vi "校准UI.vi"() -> ()   [LabVIEW 2016, in "斯坦道多参数.lvlib"]
uses:
  <vilib>/Utility/miscctls.llb/LVPointTypeDef.ctl
  <vilib>/Utility/miscctls.llb/LVPositionTypeDef.ctl
  <vilib>/ptbypt/NI_PtbyPt.lvlib
panel:
  out "溶解氧浓度值":dbl=25.0 caption="检测值：" format="%#.2f mg/L"
  out "电极状态标志":u16
  in  "恢复出厂":bool
  in  "电极系数面板":enum32{"选项卡 1"}(tab)
  out "B":dbl=25.0 caption="电极零点：" format="%#.6f"
  out "K":dbl=25.0 caption="电极系数：" format="%#.6f"
  in  "测试参数面板":enum32{"选项卡 1"}(tab)
  in  "自动盐度补偿":bool caption="自动盐度补偿："
  in  "偏移修正值":dbl=25.0 caption="偏移修正值：" format="%#_6f"
  in  "滤波次数":dbl=25.0 caption="滤波次数：" format="%#_6f"
  in  "测量量程":u16(ring)=1 caption="测量量程："
  in  "盐度":dbl=25.0 caption="盐度：" format="%#_6f"
  in  "大气压力":dbl=25.0 caption="大气压力：" format="%#_6f"
  in  "温度系数":dbl=25.0 caption="温度系数：" format="%#.6f"
  out "信号值":dbl=25.0 caption="信号值：" format="%#.2f mV"
  out "检测值":dbl=25.0 caption="检测值：" format="%#.2f"
  out "序列号":string caption="序列号："
  in  "选项卡控件 3":enum32{"选项卡 1"}(tab)
  in  "清扫间隔":u16=25 caption="清扫间隔："
  in  "清扫次数":u16=25 caption="清扫次数："
  in  "清洗":bool caption="探头清洗："
  in  "清扫模式":u16(ring)=1 caption="清扫模式：" items=["自动", "手动"]
  in  "选项卡控件 2":enum32{"选项卡 1"}(tab)
  in  "温度校准系数写入":bool
  in  "温度校准系数读取":bool
  in  "BT":dbl caption="B：" format="%#.6f"
  in  "KT":dbl=1.0 caption="K：" format="%#.6f"
  in  "实际温度":dbl=25.0 caption="校准温度：" format="%.2f ℃"
  out "当前温度":dbl caption="探头温度：" format="%.2f ℃"
  in  "校准温度":bool
  in  "选项卡控件":enum32{"选项卡 1"}(tab)
  in  "第三点确认校准":bool
  in  "第二点确认校准":bool
  in  "标液一":cluster{"标准值":dbl, "检测值":dbl, "原始值":dbl} caption="标液一：" {"原始值" format="%#_6f"; "检测值" format="%#_6f"; "标准值" format="%#.6f"}
  in  "标液二":cluster{"标准值":dbl, "检测值":dbl, "原始值":dbl} caption="标液二：" {"原始值" format="%#_6f"; "检测值" format="%#_6f"; "标准值" format="%#.6f"}
  in  "标液三":cluster{"标准值":dbl, "检测值":dbl, "原始值":dbl} caption="标液三：" {"原始值" format="%#_6f"; "检测值" format="%#_6f"; "标准值" format="%#.6f"}
  in  "标液一开始校准":bool
  in  "第一点确认校准":bool
  in  "标液二开始校准":bool
  in  "标液三开始校准":bool
  in  "显示曲线":bool
  in  "校准记录":string="校准记录\n---------------------------------------------\n序列号：\n温度值：\n标准值：\n检测值：\n原始值：\n校准时间："
  in  "校准方式":u16(ring)=1 caption="校准方式：" items=["单点校准", "两点校准", "三点校准"]
  in  "校准参数":u16(ring) caption="校准参数：" items=["pH"=0, "DO"=1, "浊度"=2, "电导率"=3, "COD"=7, "氯化物"=9, "氨氮"=10]
  # "检测值"
  # "信号值"
  # "标准值"
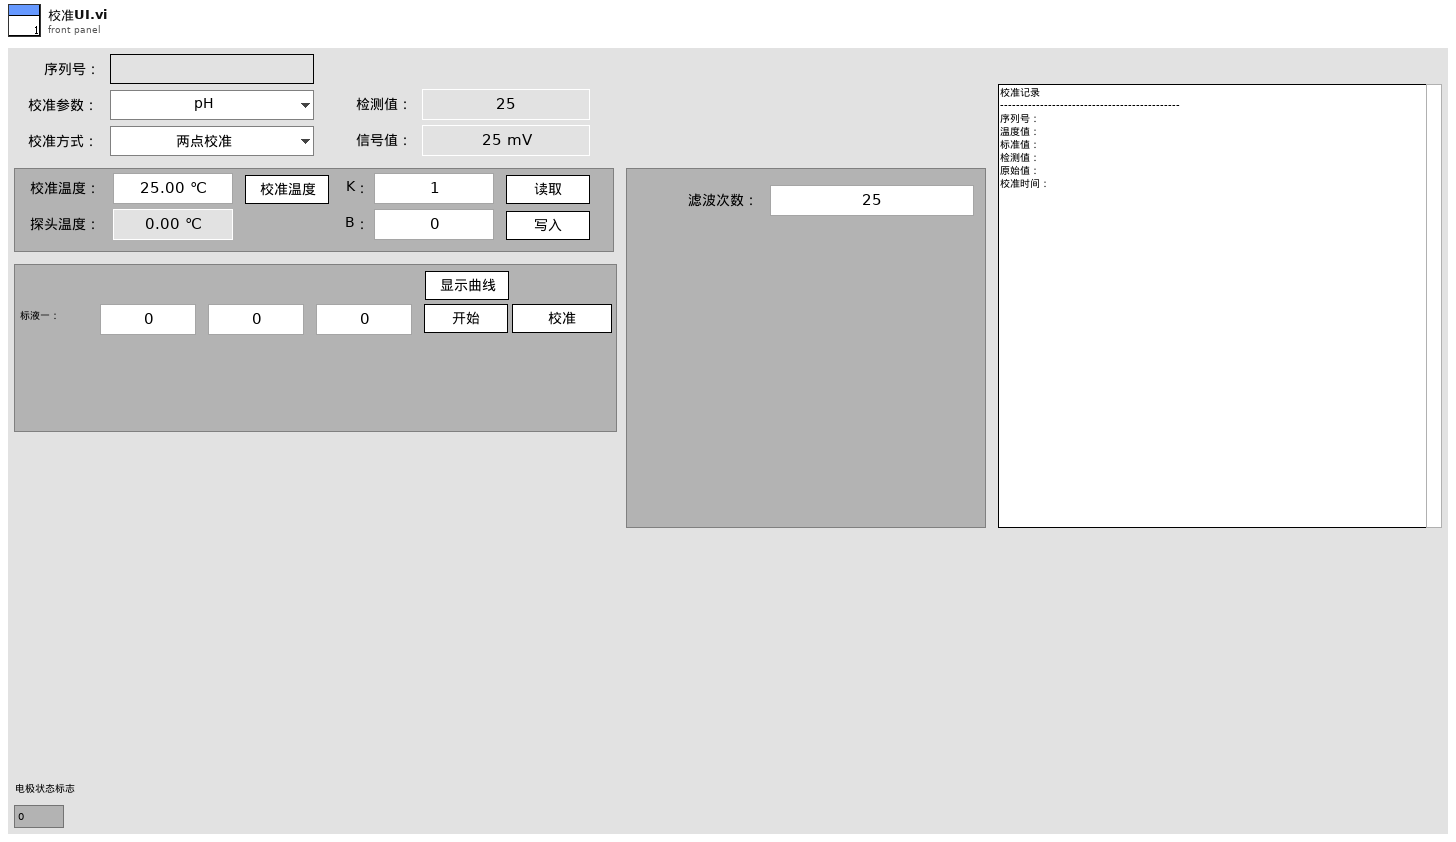
[diagram p1: front panel]
types:
  T1 = typedef "LVPointTypeDef.ctl" = cluster{"Horizontal":i16, "Vertical":i16}
  T2 = cluster{"ph":bool, "DO":bool, "Cond":bool, "Turb":bool, "叶绿素a":bool, "藻密度":bool, "ORP":bool, "COD":bool, "DO2":bool, bool, "氨氮":bool, "水中油":bool}
  T3 = typedef "斯坦道多参数.lvlib/探头类型.ctl" = enum16{"禹山", "国弘", "纳清", "STD"}
  T4 = typedef "LVStringsAndValuesArrayTypeDef_U16.ctl" = cluster{"String":string, "Value":u16}[]
  T5 = enum8{"Enabled", "Disabled", "Disabled and Grayed Out"}
  T6 = typedef "LVPositionTypeDef.ctl" = cluster{"Left":i32, "Top":i32}
  T7 = cluster{"pH":u32, "DO":u32, "Cond":u32, "Turb":u32, "叶绿素a":u32, "藻密度":u32, "ORP":u32, "COD":u32, "氯化物":u32, "氨氮":u32, "水中油":u32}
  T8 = cluster{"电极状态标志":u16, "电极型号标志":u16, "酸碱度测量值":sgl, "温度测量值":sgl, "酸碱度信号值":sgl, "温度信号值":sgl, "酸碱度偏移修正值":sgl, "温度偏移修正值":sgl, "手动温度补偿值":sgl, "酸碱度电极零点":sgl, "酸碱度电极斜率":sgl, "第1点标准值记录":sgl, "第1点信号值记录":sgl, "第1点温度值记录":sgl, "第2点标准值记录":sgl, "第2点信号值记录":sgl, "第2点温度值记录":sgl, "命令滤波设定":u16, "温度模式":enum16{"ATC", "MTC"}, "生产批次":u16, "电极序号":u16, "串口地址":u16, "串口波特率":enum16{"9600", "19200", "115200"}, "串口校验位":enum16{"NONE", "ODD", "EVEN"}, "串口停止位":enum16{"1bit", "2bit"}, "第一点标准值":sgl, "第二点标准值":sgl}
  T9 = cluster{"报警码":u16, "溶解氧数值（mg/L）":sgl, "溶解氧数据（%）":sgl, "温度数据":sgl, "溶解氧原始信号 nA":sgl, "大气压力":sgl, "盐度":sgl, "0X0009_NC":string, "产品名称":string, "序列号":string, "硬件版本":string, "软件版本":string, "通讯地址":u16, "波特率":u16, "设备类型":u16, "0X0026_NC":string, "第一点原始数据":sgl, "第一点校准数据":sgl, "第二点原始数据":sgl, "第二点校准数据":sgl, "探头校准命令":u16, "温度校准参数":sgl, "温度校准命令":u16}
  T10 = cluster{"电极状态标志":u16, "电极型号标志":u16, "溶解氧测量值":sgl, "温度测量值":sgl, "溶解氧饱和度值":sgl, "盐度补偿值":sgl, "大气压补偿值":sgl, "溶解氧偏移修正值":sgl, "温度偏移修正值":sgl, "手动温度补偿值":sgl, "溶解氧电极零点":sgl, "溶解氧电极斜率":sgl, "第1点标准值记录":sgl, "第1点信号值记录":sgl, "第1点温度值记录":sgl, "第2点标准值记录":sgl, "第2点信号值记录":sgl, "第2点温度值记录":sgl, "命令滤波设定":u16, "温度模式":enum16{"ATC", "MTC"}, "生产批次":u16, "电极序号":u16, "串口地址":u16, "串口波特率":enum16{"9600", "19200", "115200"}, "串口校验位":enum16{"NONE", "ODD", "EVEN"}, "串口停止位":enum16{"1bit", "2bit"}, "第一点标准值":sgl, "第二点标准值":sgl}
  T11 = cluster{"电极状态标志":u16, "电极型号标志":u16, "浊度测量值":sgl, "温度测量值":sgl, "浊度信号值":sgl, "浊度偏移修正值":sgl, "温度偏移修正值":sgl, "手动温度补偿值":sgl, "浊度电极零点":sgl, "浊度电极斜率":sgl, "清洁周期":u16, "命令滤波设定":u16, "温度模式":enum16{"ATC", "MTC"}, "生产批次":u16, "电极序号":u16, "串口地址":u16, "串口波特率":enum16{"9600", "19200", "115200"}, "串口校验位":enum16{"NONE", "ODD", "EVEN"}, "串口停止位":enum16{"1bit", "2bit"}, "第一点标准值":sgl, "第二点标准值":sgl, "第三点标准值":sgl}
  T12 = cluster{"报警码":u16, "浊度数值 NTU":sgl, "温度数据":sgl, "原始光强数值":u16, "量程":u16, "平均次数":u16, "清扫模式":u16, "清扫次数":u16, "清扫间隔分钟":u16, "0X000B_NC":string, "产品名称":string, "序列号":string, "硬件版本":string, "软件版本":string, "通讯地址":u16, "波特率":u16, "设备类型":u16, "0X0026_NC":string, "校准量程":u16, "第一点原始光强":u16, "第一点校准数据":sgl, "第二点原始光强":u16, "第二点校准数据":sgl, "第三点原始光强":u16, "第三点校准数据":sgl, "探头校准命令":u16, "温度校准参数":sgl, "温度校准命令":u16}
  T13 = cluster{"电极状态标志":u16, "电极型号标志":u16, "电导率测量值":sgl, "温度测量值":sgl, "电导率信号值":sgl, "温度信号值":sgl, "温度补偿系数":sgl, "电导率偏移修正值":sgl, "温度偏移修正值":sgl, "手动温度补偿值":sgl, "电导率电极零点":sgl, "电导率电极斜率":sgl, "命令滤波设定":u16, "温度模式":enum16{"ATC", "MTC"}, "生产批次":u16, "电极序号":u16, "串口地址":u16, "串口波特率":enum16{"9600", "19200", "115200"}, "串口校验位":enum16{"NONE", "ODD", "EVEN"}, "串口停止位":enum16{"1bit", "2bit"}, "第一点标准值":sgl, "第二点标准值":sgl}
  T14 = cluster{"报警码":u16, "叶绿素a":sgl, "温度数据":sgl, "原始光强数值":u16, "量程":u16, "平均次数":u16, "清扫模式":u16, "清扫次数":u16, "清扫间隔分钟":u16, "0X000B_NC":string, "产品名称":string, "序列号":string, "硬件版本":string, "软件版本":string, "通讯地址":u16, "波特率":u16, "设备类型":u16, "0X0026_NC":string, "校准量程":u16, "第一点原始光强":u16, "第一点校准数据":sgl, "第二点原始光强":u16, "第二点校准数据":sgl, "第三点原始光强":u16, "第三点校准数据":sgl, "探头校准命令":u16, "温度校准参数":sgl, "温度校准命令":u16}
  T15 = cluster{"报警码":u16, "蓝绿藻":sgl, "温度数据":sgl, "原始光强数值":u16, "量程":u16, "平均次数":u16, "清扫模式":u16, "清扫次数":u16, "清扫间隔分钟":u16, "0X000B_NC":string, "产品名称":string, "序列号":string, "硬件版本":string, "软件版本":string, "通讯地址":u16, "波特率":u16, "设备类型":u16, "0X0026_NC":string, "校准量程":u16, "第一点原始光强":u16, "第一点校准数据":sgl, "第二点原始光强":u16, "第二点校准数据":sgl, "第三点原始光强":u16, "第三点校准数据":sgl, "探头校准命令":u16, "温度校准参数":sgl, "温度校准命令":u16}
  T16 = cluster{"电极状态标志":u16, "电极型号标志":u16, "测量值":sgl, "温度测量值":sgl, "信号值":sgl, "温度信号值":sgl, "000AH_NC":sgl, "偏移修正值":sgl, "温度偏移修正值":sgl, "手动温度补偿值":sgl, "命令滤波设定":u16, "温度模式":enum16{"ATC", "MTC"}, "生产批次":u16, "传感器序号":u16, "串口地址":u16, "串口波特率":enum16{"9600", "19200", "115200"}, "串口校验位":enum16{"NONE", "ODD", "EVEN"}, "串口停止位":enum16{"1bit", "2bit"}}
  T17 = cluster{"电极状态标志":u16, "电极型号标志":u16, "COD测量值":sgl, "浊度测量值":sgl, "COD信号值":sgl, "浊度信号值":sgl, "温度测量值":sgl, "COD偏移修正值":sgl, "浊度偏移修正值":sgl, "COD水样校正值":sgl, "温度偏移修正值":sgl, "COD零点系数":sgl, "COD斜率系数":sgl, "浊度零点系数":sgl, "浊度斜率系数":sgl, "COD测值K值":sgl, "浊度测值K值":sgl, "浊度补偿COD系数值":sgl, "COD温度补偿系数值 ":sgl, "测量周期":u16, "清洗周期":u16, "命令寄存器":u16, "数字滤波设定":u16, "温度模式":enum16{"AUTO", "OFF"}, "生产批次":u16, "电极序号":u16, "串口地址":u16, "串口波特率":enum16{"9600", "19200", "115200"}, "串口校验位":enum16{"NONE", "ODD", "EVEN"}, "串口停止位":enum16{"1bit", "2bit"}, "第一点校正指令":u16, "第一点标准值":sgl, "第二点校正指令":u16, "第二点标准值":sgl, "第三点校正指令":u16, "第三点标准值":sgl, "COD吸光度":sgl, "浊度吸光度":sgl, "温度信号值":sgl}
  T18 = cluster{"电极状态标志":u16, "电极型号标志":u16, "测量值":sgl, "温度测量值":sgl, "信号值":sgl, "温度信号值":sgl, "偏移修正值":sgl, "温度偏移修正值":sgl, "手动温度补偿值":sgl, "电极零点":sgl, "电极斜率":sgl, "第1点标准值记录":sgl, "第1点信号值记录":sgl, "第1点温度值记录":sgl, "第2点标准值记录":sgl, "第2点信号值记录":sgl, "第2点温度值记录":sgl, "命令滤波设定":u16, "温度模式":enum16{"ATC", "MTC"}, "生产批次":u16, "电极序号":u16, "串口地址":u16, "串口波特率":enum16{"9600", "19200", "115200"}, "串口校验位":enum16{"NONE", "ODD", "EVEN"}, "串口停止位":enum16{"1bit", "2bit"}, "第一点标准值":sgl, "第二点标准值":sgl}
  T19 = cluster{"电极状态标志":u16, "电极型号标志":u16, "测量值":sgl, "温度测量值":sgl, "信号值":sgl, "水中油B值":sgl, "温度B值":sgl, "水中油零点系数":sgl, "水中油斜率系数":sgl, "水中油K值":sgl, "空白电位值":sgl, "温度信号值":sgl, "温度补偿系数":sgl, "测量档位":u16, "清洁周期":u16, "命令寄存器":u16, "数位滤波设定":u16, "温度模式":enum16{"ATC", "MTC"}, "生产批次":u16, "电极序号":u16, "串口地址":u16, "串口波特率":enum16{"9600", "19200", "115200"}, "串口校验位":enum16{"NONE", "ODD", "EVEN"}, "串口停止位":enum16{"1bit", "2bit"}, "第一点校正指令":u16, "第一点标准值":sgl, "第二点校正指令":u16, "第二点标准值":sgl, "第三点校正指令":u16, "第三点标准值":sgl}
  T20 = enum16{"null", "pH", "DO", "浊度", "电导率", "叶绿素a", "DO2", "藻密度"}
  T21 = enum16{"null", "pH", "DO", "浊度", "电导率", "叶绿素a", "藻密度"}
  T22 = cluster{"禁用":enum8{"Enabled", "Disabled", "Disabled and Grayed Out"}, "禁用 2":enum8{"Enabled", "Disabled", "Disabled and Grayed Out"}, "禁用 3":enum8{"Enabled", "Disabled", "Disabled and Grayed Out"}}
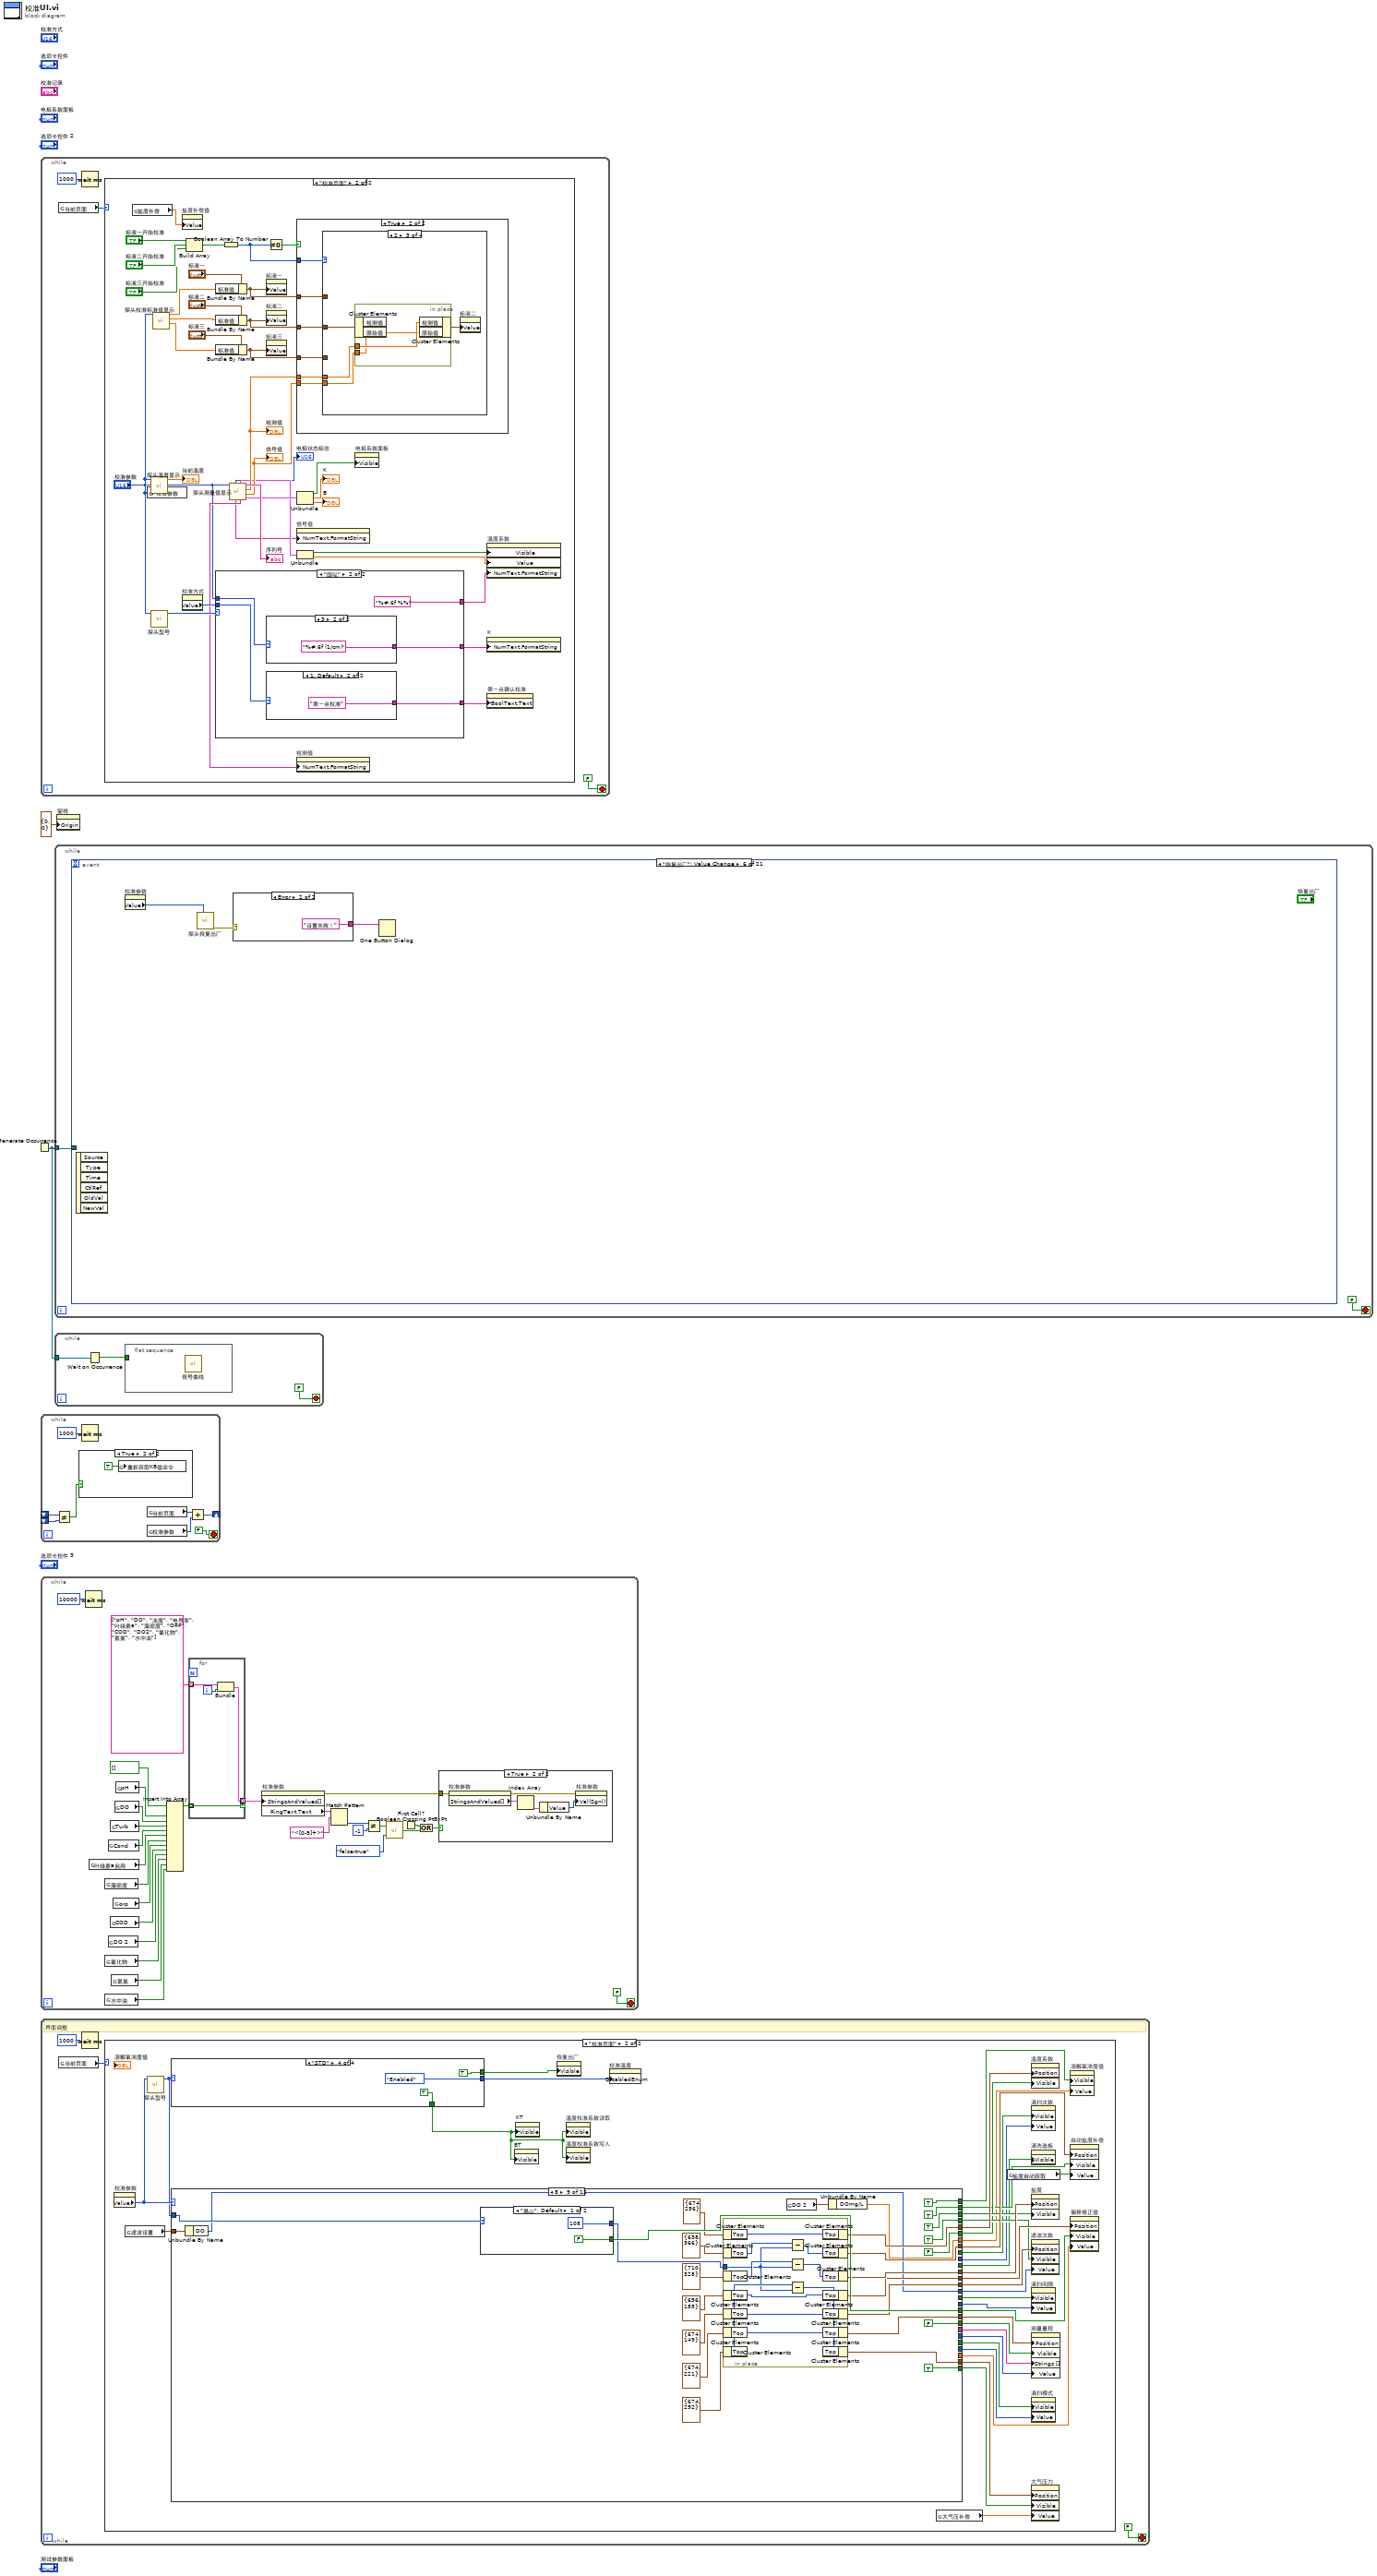
[diagram p0: block diagram]
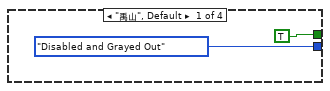
[diagram p4: hidden frame]
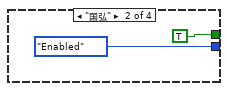
[diagram p5: hidden frame]
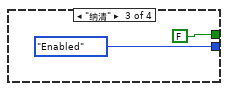
[diagram p6: hidden frame]
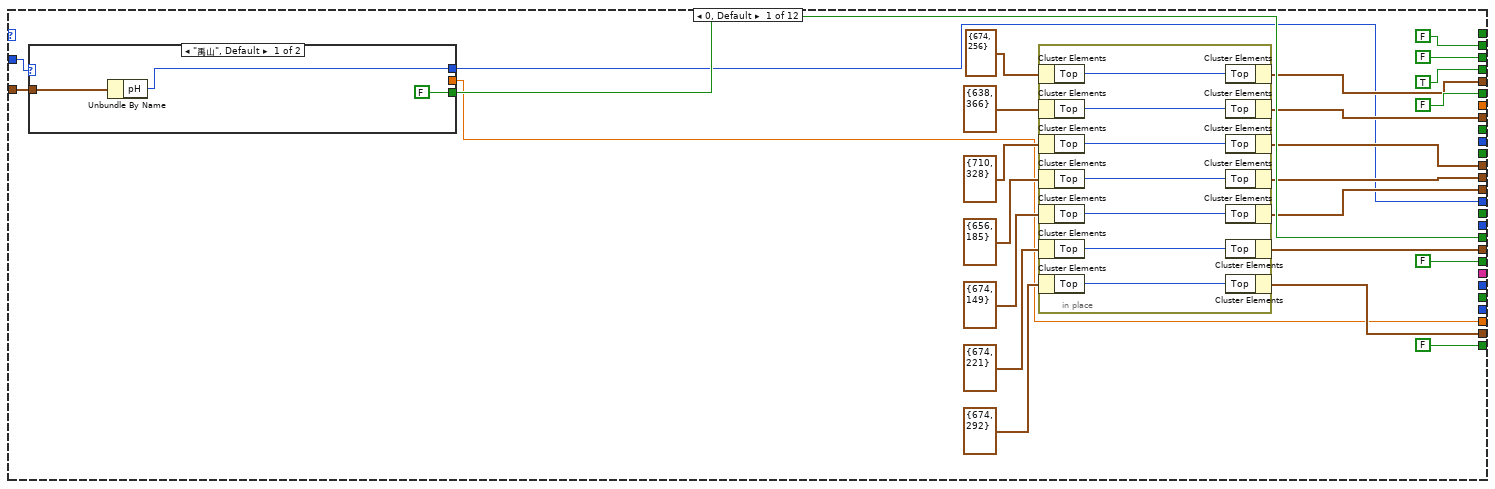
[diagram p7: hidden frame]
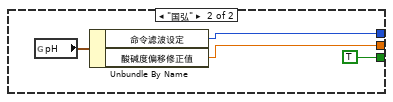
[diagram p8: hidden frame]
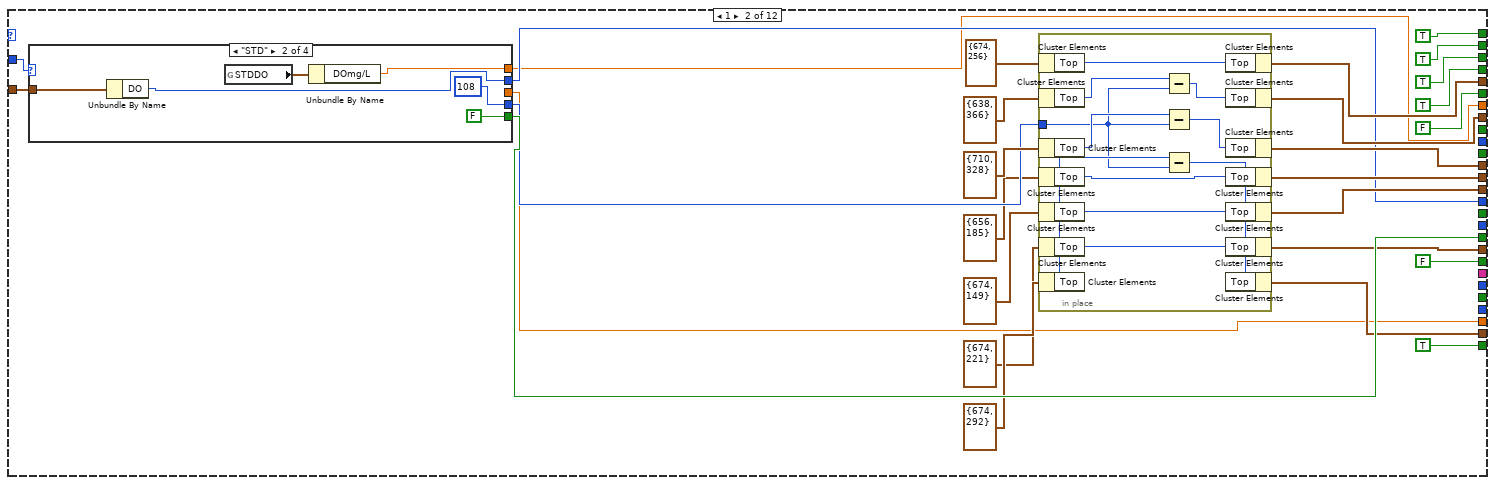
[diagram p9: hidden frame]
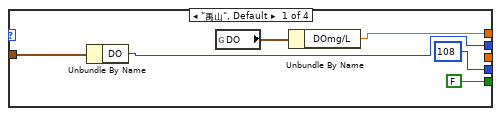
[diagram p10: hidden frame]
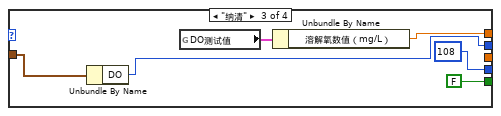
[diagram p11: hidden frame]
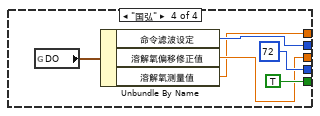
[diagram p12: hidden frame]
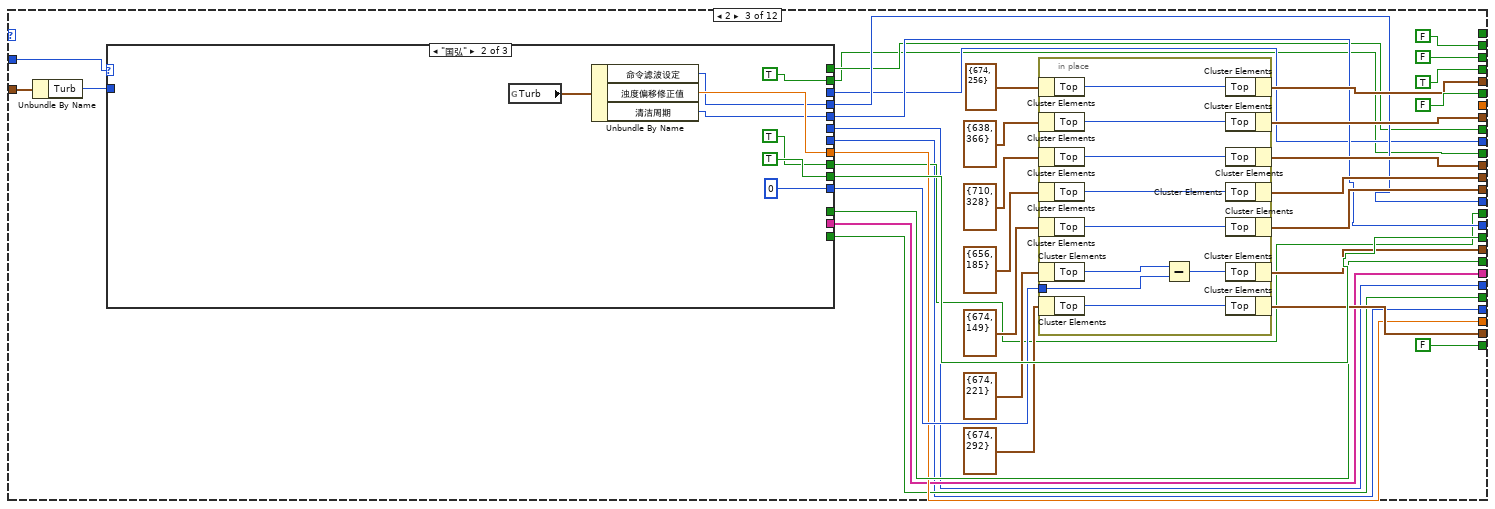
[diagram p13: hidden frame]
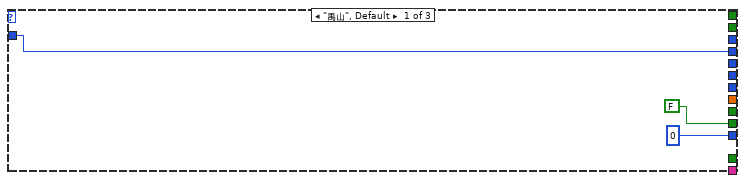
[diagram p14: hidden frame]
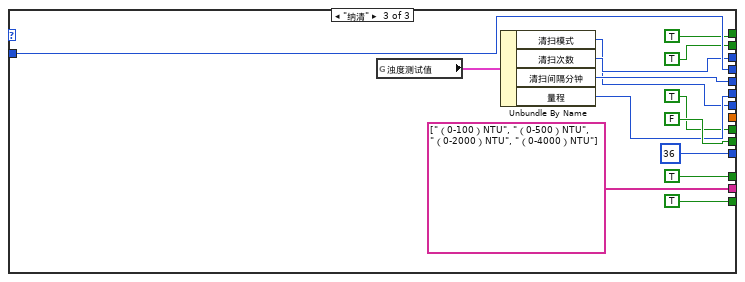
[diagram p15: hidden frame]
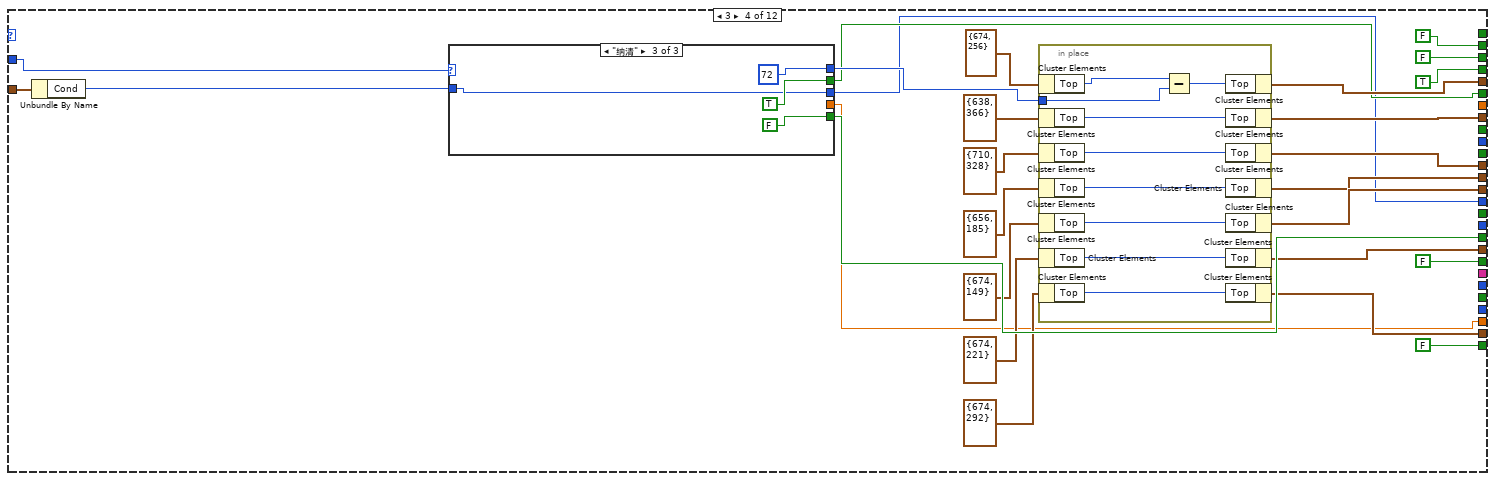
[diagram p16: hidden frame]
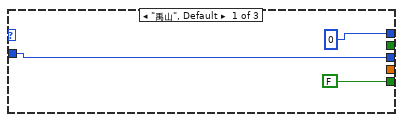
[diagram p17: hidden frame]
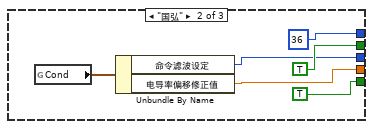
[diagram p18: hidden frame]
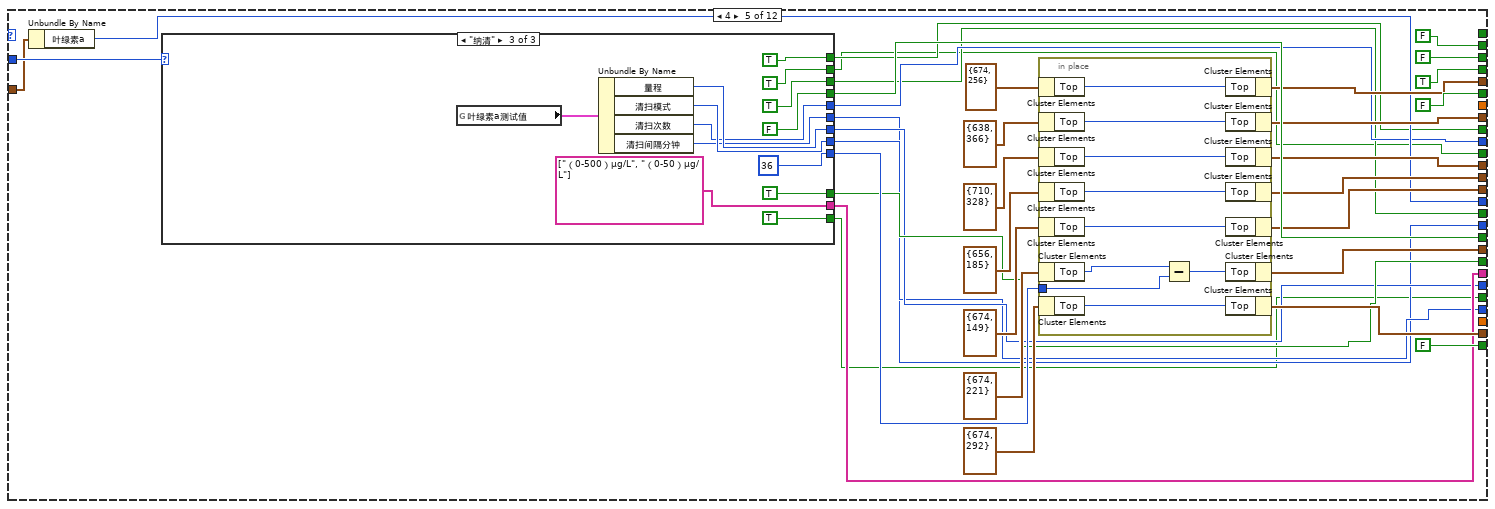
[diagram p19: hidden frame]
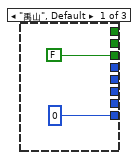
[diagram p20: hidden frame]
diagram:
  n1 = Generate Occurrence() -> (w1:refnum<k4>)
  n2 = while {
    stop <- FALSE stop-if-true
    n3 = global read "多参数全局变量.vi" "当前页面"() -> (w3:enum16{"主页面", "参数页面", "校准页面"})
    n4 = Wait (ms)(milliseconds to wait=u32 1000 ("等待时间（毫秒）")) -> ()  [unwired: 1 out]
    n5 = case shown="\"校准页面\"" w3 {
      frame "主页面", Default {
        n6 = global write "多参数全局变量.vi" "校准运行状态"(T2 {"ph"=FALSE, "DO"=FALSE, "Cond"=FALSE, "Turb"=FALSE, "叶绿素a"=FALSE, "藻密度"=FALSE, "ORP"=FALSE, "COD"=FALSE, "DO2"=FALSE, FALSE, "氨氮"=FALSE, "水中油"=FALSE} ("校准运行状态")) -> ()
      }
      frame "校准页面" {
        n7 = global read "断电保存变量.vi" "盐度补偿"() -> (w29:dbl)
        n8 = global write "多参数全局变量.vi" "校准参数"("校准参数") -> ()
        n9 = call "探头温度显示.vi"("校准参数"="校准参数") -> ("温度数据"=→"当前温度":sgl)  [unwired: 9 in, 1 out]
        n10 = call "探头型号.vi"("校准参数"="校准参数") -> ("探头型号"=w24:T3)  [unwired: 8 in, 2 out]
        n11 = call "探头校准标准值显示.vi"("校准参数"="校准参数") -> ("标液三"=w42:sgl, "标液二"=w41:sgl, "标液一"=w40:sgl)  [unwired: 8 in]
        n12 = property on="盐度补偿值" class="DigNum (strict)"("Value"=w29) -> ()  [unwired: 2 in, 2 out]
        n13 = property on="校准方式" class="Ring (strict)"() -> ("Value"=w22:u16)  [unwired: 2 in, 2 out]
        n14 = Build Array("标液一开始校准", "标液二开始校准", "标液三开始校准") -> (w10:bool[])
        n15 = Bundle By Name(cluster="标液一", "标准值"=w40) -> (w36:cluster{"标准值":dbl, "检测值":dbl, "原始值":dbl})
        n16 = Bundle By Name(cluster="标液二", "标准值"=w41) -> (w35:cluster{"标准值":dbl, "检测值":dbl, "原始值":dbl})
        n17 = Bundle By Name(cluster="标液三", "标准值"=w42) -> (w34:cluster{"标准值":dbl, "检测值":dbl, "原始值":dbl})
        n18 = case shown="\"国弘\"" w24 {
          tunnel: ["校准" w50] -> w23
          tunnel: w22 -> [_ w49]
          tunnel: "校准参数" -> [_ w48]
          tunnel: ["%#.6f" ("数值文本.格式字符串") w47] -> w15
          tunnel: ["%#.6f" ("数值文本.格式字符串") "%#.6f %%" ("数值文本.格式字符串")] -> w14
          frame "禹山", Default {
          }
          frame "国弘" {
            n19 = case shown="3" w48 {
              tunnel: ["%#.6f" ("数值文本.格式字符串") "%#.6f (1/cm)" ("数值文本.格式字符串")] -> w47
              frame 0, Default {
              }
              frame 3 {
              }
            }
            n20 = case shown="1, Default" w49 {
              tunnel: ["校准" "第一点校准"] -> w50
              frame 0 {
              }
              frame 1, Default {
              }
            }
          }
        }
        n21 = Boolean Array To Number(Boolean array=w10) -> (number=w8:u32)
        n22 = call "探头测量值显示.vi"("校准参数"="校准参数") -> ("线性系数"=w28:cluster{bool, "K":sgl, "B":sgl}, "信号值"=w30:sgl, "检测值"=w31:sgl, "序列号"=→"序列号":string, "检测值.格式字符串"=w21:string, "温度补偿系数"=w20:cluster{bool, "温度补偿系数":sgl}, "信号值.格式字符串"=w16:string, "电极状态标志"=→"电极状态标志":u16)  [unwired: 3 in]
        "检测值" <- w31
        "信号值" <- w30
        n23 = property on="标液一" class="Clust (strict)"("Value"=w36) -> ()  [unwired: 2 in, 2 out]
        n24 = property on="标液二" class="Clust (strict)"("Value"=w35) -> ()  [unwired: 2 in, 2 out]
        n25 = property on="标液三" class="Clust (strict)"("Value"=w34) -> ()  [unwired: 2 in, 2 out]
        n26 = Not Equal To 0?(x=w8) -> (x != 0?=w9:bool)
        n27 = case shown="True" w9 {
          tunnel: w36 -> [_ w60]
          tunnel: w35 -> [_ w59]
          tunnel: w34 -> [_ w58]
          tunnel: w30 -> [_ w57]
          tunnel: w31 -> [_ w56]
          tunnel: w8 -> [_ w55]
          frame False {
          }
          frame True {
            n28 = case shown="2" w55 {
              tunnel: w56 -> [_ w63 w70 w76]
              tunnel: w57 -> [_ w62 w69 w75]
              tunnel: w60 -> [_ w64 _ _]
              tunnel: w59 -> [_ _ w67 _]
              tunnel: w58 -> [_ _ _ w73]
              frame Default {
              }
              frame 1 {
                n29 = in-place {
                  in-place-border: w63 -> [w66]
                  in-place-border: w62 -> [w65]
                  n30 = in-place-cluster #1(w64) -> ()  [unwired: 2 out]
                  n31 = in-place-cluster #1("检测值"=w66, "原始值"=w65) -> (w61:cluster{"标准值":dbl, "检测值":dbl, "原始值":dbl})
                }
                n32 = property on="标液一" class="Clust (strict)"("Value"=w61) -> ()  [unwired: 2 in, 2 out]
              }
              frame 2 {
                n33 = in-place {
                  in-place-border: w70 -> [w72]
                  in-place-border: w69 -> [w71]
                  n34 = in-place-cluster #2(w67) -> ()  [unwired: 2 out]
                  n35 = in-place-cluster #2("检测值"=w72, "原始值"=w71) -> (w68:cluster{"标准值":dbl, "检测值":dbl, "原始值":dbl})
                }
                n36 = property on="标液二" class="Clust (strict)"("Value"=w68) -> ()  [unwired: 2 in, 2 out]
              }
              frame 4 {
                n37 = in-place {
                  in-place-border: w76 -> [w78]
                  in-place-border: w75 -> [w77]
                  n38 = in-place-cluster #3(w73) -> ()  [unwired: 2 out]
                  n39 = in-place-cluster #3("检测值"=w78, "原始值"=w77) -> (w74:cluster{"标准值":dbl, "检测值":dbl, "原始值":dbl})
                }
                n40 = property on="标液三" class="Clust (strict)"("Value"=w74) -> ()  [unwired: 2 in, 2 out]
              }
            }
          }
        }
        n41 = Unbundle(w28) -> (w27:bool, "K"=→"K":sgl, "B"=→"B":sgl)
        n42 = property on="信号值" class="DigNum (strict)"("NumText.FormatString"=w16) -> ()  [unwired: 2 in, 2 out]
        n43 = Unbundle(w20) -> (w19:bool, "温度补偿系数"=w18:sgl)
        n44 = property on="检测值" class="DigNum (strict)"("NumText.FormatString"=w21) -> ()  [unwired: 2 in, 2 out]
        n45 = property on="电极系数面板" class="TabCtl (strict)"("Visible"=w27) -> ()  [unwired: 2 in, 2 out]
        n46 = property on="温度系数" class="DigNum (strict)"("Visible"=w19, "Value"=w18, "NumText.FormatString"=w14) -> ()  [unwired: 2 in, 2 out]
        n47 = property on="K" class="DigNum (strict)"("NumText.FormatString"=w15) -> ()  [unwired: 2 in, 2 out]
        n48 = property on="第一点确认校准" class="Bool"("BoolText.Text"=w23) -> ()  [unwired: 2 in, 2 out]
      }
    }
  }
  n49 = while {
    shift-right: [w82] -> _
    shift-left: _ -> [w81]
    shift-left: _ -> [w80]
    stop <- FALSE stop-if-true
    n50 = Not Equal?(x=w81, y=w80) -> (x != y?=w79:bool)
    n51 = case shown="True" w79 {
      frame False {
      }
      frame True {
        n52 = global write "多参数全局变量.vi" "重新获取KB值命令"(TRUE ("重新获取KB值命令")) -> ()
      }
    }
    n53 = Wait (ms)(milliseconds to wait=u32 1000 ("等待时间（毫秒）")) -> ()  [unwired: 1 out]
    n54 = global read "多参数全局变量.vi" "当前页面"() -> (w83:enum16{"主页面", "参数页面", "校准页面"})
    n55 = global read "多参数全局变量.vi" "校准参数"() -> (w84:u16)
    n56 = Add(x=w83, y=w84) -> (x+y=w82:u16)
  }
  n57 = while {
    stop <- FALSE stop-if-true
    n58 = Wait (ms)(milliseconds to wait=u32 10000 ("等待时间（毫秒）")) -> ()  [unwired: 1 out]
    n59 = global read "断电保存变量.vi" "叶绿素a启用"() -> (w110:bool)
    n60 = global read "断电保存变量.vi" "藻密度"() -> (w109:bool)
    n61 = global read "断电保存变量.vi" "氯化物"() -> (w89:bool)
    n62 = global read "断电保存变量.vi" "水中油"() -> (w88:bool)
    n63 = global read "断电保存变量.vi" "Cond"() -> (w111:bool)
    n64 = global read "断电保存变量.vi" "DO 2"() -> (w90:bool)
    n65 = global read "断电保存变量.vi" "Turb"() -> (w112:bool)
    n66 = global read "断电保存变量.vi" "COD"() -> (w91:bool)
    n67 = global read "断电保存变量.vi" "氨氮"() -> (w92:bool)
    n68 = global read "断电保存变量.vi" "orp"() -> (w108:bool)
    n69 = global read "断电保存变量.vi" "DO"() -> (w113:bool)
    n70 = global read "断电保存变量.vi" "pH"() -> (w115:bool)
    n71 = Insert Into Array(array=bool[] [] ("数组"), new element #1=w115, new element #2=w113, new element #3=w112, new element #4=w111, new element #5=w110, new element #6=w109, new element #7=w108, new element #8=w91, new element #9=w90, new element #10=w89, new element #11=w92, new element #12=w88) -> (w105:bool[])  [unwired: 1 in]
    n72 = for {
      tunnel: w105 -> [w121] mode=indexing
      tunnel: string[] ["pH", "DO", "浊度", "电导率", "叶绿素a", "藻密度", "ORP", "COD", "DO2", "氯化物", "氨氮", "水中油"] ("字符串[]") -> [w123] mode=indexing
      tunnel: [w122] -> w102 mode=indexing if=w121
      i -> [w124]
      n73 = Bundle(w123, w124) -> (w122:cluster{string, i32})  [unwired: 1 in]
    }
    n74 = property on="校准参数" class="Ring (strict)"("StringsAndValues[]"=w102) -> (error out=w103:errorcluster, "RingText.Text"=w101:string)  [unwired: 2 in, 1 out]
    n75 = Match Pattern(string=w101, regular expression="<[0-9]+>" ("正则表达式")) -> (offset past match=w99:i32)  [unwired: 1 in, 3 out]
    n76 = Not Equal?(x=w99, y=-1) -> (x != y?=w97:bool)
    n77 = call <vilib>:"Boolean Crossing PtByPt.vi"("direction"=enum16{"either", "false-true", "true-false"}."false-true", "input"=w97) -> ("crossing"=w94:bool)  [unwired: 1 in]
    n78 = First Call?() -> (First Call?: T/F=w95:bool)
    n79 = Or(x=w95, y=w94) -> (x .or. y?=w96:bool)
    n80 = case shown="True" w96 {
      tunnel: w103 -> [_ w120]
      frame False {
      }
      frame True {
        n81 = property on="校准参数" class="Ring (strict)"(error in=w120) -> (error out=w119:errorcluster, "StringsAndValues[]"=w118:T4)  [unwired: 1 in, 1 out]
        n82 = Index Array(array=w118) -> (element=w117:cluster{"String":string, "Value":u16})  [unwired: 1 in]
        n83 = Unbundle By Name(w117) -> ("Value"=w116:u16)
        n84 = property on="校准参数" class="Ring (strict)"(error in=w119, "Val(Sgnl)"=w116) -> ()  [unwired: 1 in, 2 out]
      }
    }
  }
  n85 = while {
    stop <- FALSE stop-if-true
    # "界面调整"
    n86 = global read "多参数全局变量.vi" "当前页面"() -> (w126:enum16{"主页面", "参数页面", "校准页面"})
    n87 = Wait (ms)(milliseconds to wait=u32 1000 ("等待时间（毫秒）")) -> ()  [unwired: 1 out]
    n88 = case shown="\"校准页面\"" w126 {
      frame "主页面", Default {
      }
      frame "校准页面" {
        n89 = property on="校准参数" class="Ring (strict)"() -> ("Value"=w161:u16)  [unwired: 2 in, 2 out]
        n90 = global read "断电保存变量.vi" "滤波设置"() -> (w143:T7)
        n91 = call "探头型号.vi"("校准参数"=w161) -> ("探头型号"=w131:T3)  [unwired: 8 in, 2 out]
        n92 = case shown="\"STD\"" w131 {
          tunnel: [TRUE TRUE FALSE TRUE] -> w130
          tunnel: [T5."Disabled and Grayed Out" ("禁用") T5."Enabled" ("禁用") T5."Enabled" ("禁用") T5."Enabled" ("禁用")] -> w129
          tunnel: [_ _ _ TRUE] -> w128
          frame "禹山", Default {
          }
          frame "国弘" {
          }
          frame "纳清" {
          }
          frame "STD" {
          }
        }
        n93 = case shown="8" w161 {
          tunnel: [w181 w222 w294 w356 w411 w471 w523 w561 w594 w635 w665 w699] -> w162
          tunnel: w131 -> [w189 w231 w303 w365 w420 w480 w531 _ w603 _ _ _]
          tunnel: [w179 w220 w292 w354 w409 w469 w521 w559 w592 w633 w663 w697] -> w160
          tunnel: [w177 w218 w290 w352 w407 w467 w519 w557 w590 w631 w661 w695] -> w159
          tunnel: [w175 w216 w288 w350 w405 w465 w517 w555 w588 w629 w659 w693] -> w158
          tunnel: [w183 w224 w296 w358 w413 w473 w525 w563 w596 w637 w667 w701] -> w157
          tunnel: [w185 w227 w299 w361 w416 w476 w527 w565 w599 w639 w669 w704] -> w156
          tunnel: [w184 w225 w297 w359 w414 w474 w526 w564 w597 w638 w668 w702] -> w155
          tunnel: [TRUE TRUE TRUE TRUE TRUE TRUE TRUE TRUE TRUE TRUE TRUE TRUE] -> w154
          tunnel: [FALSE FALSE w287 FALSE w404 w464 FALSE FALSE FALSE FALSE FALSE _] -> w153
          tunnel: [FALSE TRUE FALSE FALSE FALSE FALSE FALSE FALSE TRUE FALSE FALSE FALSE] -> w152
          tunnel: [FALSE FALSE FALSE w348 FALSE FALSE FALSE FALSE FALSE FALSE FALSE FALSE] -> w151
          tunnel: [w192 w234 w306 w368 w423 w483 w534 TRUE w606 TRUE FALSE TRUE] -> w150
          tunnel: [FALSE TRUE FALSE FALSE FALSE FALSE FALSE FALSE TRUE FALSE FALSE FALSE] -> w149
          tunnel: [FALSE TRUE FALSE FALSE FALSE FALSE FALSE FALSE TRUE FALSE FALSE FALSE] -> w148
          tunnel: [w174 w214 w285 w345 w402 w462 w515 w554 w586 w628 w658 w691] -> w145
          tunnel: [w173 w213 w286 w344 _ _ w516 w553 _ w627 _ w692] -> w144
          tunnel: w143 -> [w172 w215 w284 w347 w403 w463 w514 _ w587 _ w657 _]
          tunnel: [_ _ w282 _ w401 w461 _ _ _ _ _ _] -> w142
          tunnel: [_ _ w281 _ w400 w460 _ _ _ _ _ _] -> w141
          tunnel: [_ _ w280 _ w397 w456 _ _ _ _ _ w690] -> w140
          tunnel: [_ _ w279 _ w394 w454 _ _ _ _ _ TRUE] -> w139
          tunnel: [_ _ w278 _ w395 w453 _ _ _ _ _ _] -> w138
          tunnel: [_ _ w277 _ w396 w455 _ _ _ _ _ _] -> w137
          tunnel: [_ _ w276 _ w398 w457 _ _ _ _ _ _] -> w136
          tunnel: [_ _ w275 _ w399 w458 _ _ _ _ _ _] -> w135
          tunnel: [_ _ w274 _ w393 w459 _ _ _ _ _ TRUE] -> w134
          tunnel: [_ w212 _ _ _ _ _ _ w584 _ _ _] -> w132
          tunnel: [_ TRUE _ _ _ _ _ _ TRUE _ _ _] -> w133
          frame 0, Default {
            n94 = case shown="\"禹山\", Default" w189 {
              tunnel: [FALSE TRUE] -> w192
              tunnel: [w204 w208] -> w174
              tunnel: [_ w207] -> w173
              tunnel: w172 -> [w205 _]
              frame "禹山", Default {
                n95 = Unbundle By Name(w205) -> ("pH"=w204:u32)
              }
              frame "国弘" {
                n96 = global read "国弘过程全局变量.vi" "pH"() -> (w209:T8)
                n97 = Unbundle By Name(w209) -> ("命令滤波设定"=w208:u16, "酸碱度偏移修正值"=w207:sgl)
              }
            }
            n98 = in-place {
              n99 = in-place-cluster #4(T6 {"Left"=674, "Top"=256} ("位置 4")) -> ("Top"=w201:i32)
              n100 = in-place-cluster #5(T6 {"Left"=638, "Top"=366} ("位置 7")) -> ("Top"=w197:i32)
              n101 = in-place-cluster #6(T6 {"Left"=710, "Top"=328} ("位置 6")) -> ("Top"=w198:i32)
              n102 = in-place-cluster #7(T6 {"Left"=656, "Top"=185} ("位置 2")) -> ("Top"=w202:i32)
              n103 = in-place-cluster #8(T6 {"Left"=674, "Top"=149} ("位置")) -> ("Top"=w203:i32)
              n104 = in-place-cluster #9(T6 {"Left"=674, "Top"=221} ("位置 3")) -> ("Top"=w200:i32)
              n105 = in-place-cluster #10(T6 {"Left"=674, "Top"=292} ("位置 5")) -> ("Top"=w199:i32)
              n106 = in-place-cluster #4("Top"=w201) -> (w175:T6)
              n107 = in-place-cluster #5("Top"=w197) -> (w184:T6)
              n108 = in-place-cluster #6("Top"=w198) -> (w185:T6)
              n109 = in-place-cluster #7("Top"=w202) -> (w179:T6)
              n110 = in-place-cluster #8("Top"=w203) -> (w181:T6)
              n111 = in-place-cluster #9("Top"=w200) -> (w177:T6)
              n112 = in-place-cluster #10("Top"=w199) -> (w183:T6)
            }
          }
          frame 1 {
            n113 = case shown="\"STD\"" w231 {
              tunnel: [FALSE FALSE FALSE TRUE] -> w234
              tunnel: [108 ("y") 108 ("y") 108 ("y") 72 ("y")] -> w226
              tunnel: w215 -> [w253 w259 w265 _]
              tunnel: [w252 w258 w264 w269] -> w214
              tunnel: [_ _ _ w270] -> w213
              tunnel: [w250 w256 w262 w268] -> w212
              frame "禹山", Default {
                n114 = Unbundle By Name(w253) -> ("DO"=w252:u32)
                n115 = global read "禹山过程全局变量.vi" "DO"() -> (w251:cluster{"温度测量值":sgl, "DO%":sgl, "DOmg/L":sgl})
                n116 = Unbundle By Name(w251) -> ("DOmg/L"=w250:sgl)
              }
              frame "STD" {
                n117 = Unbundle By Name(w259) -> ("DO"=w258:u32)
                n118 = global read "禹山过程全局变量.vi" "STDDO"() -> (w257:cluster{"温度测量值":sgl, "DO%":sgl, "DOmg/L":sgl})
                n119 = Unbundle By Name(w257) -> ("DOmg/L"=w256:sgl)
              }
              frame "纳清" {
                n120 = Unbundle By Name(w265) -> ("DO"=w264:u32)
                n121 = global read "纳清过程全局变量.vi" "DO测试值"() -> (w263:T9)
                n122 = Unbundle By Name(w263) -> ("溶解氧数值（mg/L）"=w262:sgl)
              }
              frame "国弘" {
                n123 = global read "国弘过程全局变量.vi" "DO"() -> (w271:T10)
                n124 = Unbundle By Name(w271) -> ("命令滤波设定"=w269:u16, "溶解氧偏移修正值"=w270:sgl, "溶解氧测量值"=w268:sgl)
              }
            }
            n125 = in-place {
              in-place-border: w226 -> [w243]
              n126 = in-place-cluster #11(T6 {"Left"=674, "Top"=256} ("位置 4")) -> ("Top"=w240:i32)
              n127 = in-place-cluster #12(T6 {"Left"=638, "Top"=366} ("位置 7")) -> ("Top"=w247:i32)
              n128 = in-place-cluster #13(T6 {"Left"=710, "Top"=328} ("位置 6")) -> ("Top"=w249:i32)
              n129 = in-place-cluster #14(T6 {"Left"=656, "Top"=185} ("位置 2")) -> ("Top"=w241:i32)
              n130 = in-place-cluster #15(T6 {"Left"=674, "Top"=149} ("位置")) -> ("Top"=w242:i32)
              n131 = in-place-cluster #16(T6 {"Left"=674, "Top"=221} ("位置 3")) -> ("Top"=w239:i32)
              n132 = in-place-cluster #17(T6 {"Left"=674, "Top"=292} ("位置 5")) -> ("Top"=w245:i32)
              n133 = Subtract(x=w247, y=w243) -> (x-y=w246:i32)
              n134 = Subtract(x=w249, y=w243) -> (x-y=w248:i32)
              n135 = Subtract(x=w245, y=w243) -> (x-y=w244:i32)
              n136 = in-place-cluster #11("Top"=w240) -> (w216:T6)
              n137 = in-place-cluster #12("Top"=w246) -> (w225:T6)
              n138 = in-place-cluster #13("Top"=w248) -> (w227:T6)
              n139 = in-place-cluster #14("Top"=w241) -> (w220:T6)
              n140 = in-place-cluster #15("Top"=w242) -> (w222:T6)
              n141 = in-place-cluster #16("Top"=w239) -> (w218:T6)
              n142 = in-place-cluster #17("Top"=w244) -> (w224:T6)
            }
          }
          frame 2 {
            n143 = Unbundle By Name(w284) -> ("Turb"=w283:u32)
            n144 = case shown="\"国弘\"" w303 {
              tunnel: [FALSE TRUE FALSE] -> w306
              tunnel: [0 ("y") 0 ("y") 36 ("y")] -> w298
              tunnel: [_ _ TRUE] -> w287
              tunnel: [_ w326 _] -> w286
              tunnel: [w319 w325 w340] -> w285
              tunnel: w283 -> [w319 _ w340]
              tunnel: [_ _ string[] ["（0-100）NTU", "（0-500）NTU", "（0-2000）NTU", "（0-4000）NTU"]] -> w282
              tunnel: [_ _ w337] -> w281
              tunnel: [_ w324 w335] -> w280
              tunnel: [_ TRUE TRUE] -> w279
              tunnel: [_ _ TRUE] -> w278
              tunnel: [_ _ TRUE] -> w277
              tunnel: [_ _ w332] -> w276
              tunnel: [_ _ w331] -> w275
              tunnel: [_ TRUE TRUE] -> w274
              frame "禹山", Default {
              }
              frame "国弘" {
                n145 = global read "国弘过程全局变量.vi" "Turb"() -> (w327:T11)
                n146 = Unbundle By Name(w327) -> ("命令滤波设定"=w325:u16, "浊度偏移修正值"=w326:sgl, "清洁周期"=w324:u16)
              }
              frame "纳清" {
                n147 = global read "纳清过程全局变量.vi" "浊度测试值"() -> (w338:T12)
                n148 = Unbundle By Name(w338) -> ("清扫模式"=w331:u16, "清扫次数"=w332:u16, "清扫间隔分钟"=w335:u16, "量程"=w337:u16)
              }
            }
            n149 = in-place {
              in-place-border: w298 -> [w310]
              n150 = in-place-cluster #18(T6 {"Left"=674, "Top"=256} ("位置 4")) -> ("Top"=w316:i32)
              n151 = in-place-cluster #19(T6 {"Left"=638, "Top"=366} ("位置 7")) -> ("Top"=w313:i32)
              n152 = in-place-cluster #20(T6 {"Left"=710, "Top"=328} ("位置 6")) -> ("Top"=w312:i32)
              n153 = in-place-cluster #21(T6 {"Left"=656, "Top"=185} ("位置 2")) -> ("Top"=w317:i32)
              n154 = in-place-cluster #22(T6 {"Left"=674, "Top"=149} ("位置")) -> ("Top"=w318:i32)
              n155 = in-place-cluster #23(T6 {"Left"=674, "Top"=221} ("位置 3")) -> ("Top"=w315:i32)
              n156 = in-place-cluster #24(T6 {"Left"=674, "Top"=292} ("位置 5")) -> ("Top"=w314:i32)
              n157 = Subtract(x=w315, y=w310) -> (x-y=w311:i32)
              n158 = in-place-cluster #18("Top"=w316) -> (w288:T6)
              n159 = in-place-cluster #19("Top"=w313) -> (w297:T6)
              n160 = in-place-cluster #20("Top"=w312) -> (w299:T6)
              n161 = in-place-cluster #21("Top"=w317) -> (w292:T6)
              n162 = in-place-cluster #22("Top"=w318) -> (w294:T6)
              n163 = in-place-cluster #23("Top"=w311) -> (w290:T6)
              n164 = in-place-cluster #24("Top"=w314) -> (w296:T6)
            }
          }
          frame 3 {
            n165 = Unbundle By Name(w347) -> ("Cond"=w346:u32)
            n166 = case shown="\"纳清\"" w365 {
              tunnel: [FALSE TRUE FALSE] -> w368
              tunnel: [0 ("y") 36 ("y") 72 ("y")] -> w360
              tunnel: [_ TRUE TRUE] -> w348
              tunnel: w346 -> [w380 _ w389]
              tunnel: [w380 w383 w389] -> w345
              tunnel: [_ w384 _] -> w344
              frame "禹山", Default {
              }
              frame "国弘" {
                n167 = global read "国弘过程全局变量.vi" "Cond"() -> (w385:T13)
                n168 = Unbundle By Name(w385) -> ("命令滤波设定"=w383:u16, "电导率偏移修正值"=w384:sgl)
              }
              frame "纳清" {
              }
            }
            n169 = in-place {
              in-place-border: w360 -> [w372]
              n170 = in-place-cluster #25(T6 {"Left"=674, "Top"=256} ("位置 4")) -> ("Top"=w377:i32)
              n171 = in-place-cluster #26(T6 {"Left"=638, "Top"=366} ("位置 7")) -> ("Top"=w375:i32)
              n172 = in-place-cluster #27(T6 {"Left"=710, "Top"=328} ("位置 6")) -> ("Top"=w374:i32)
              n173 = in-place-cluster #28(T6 {"Left"=656, "Top"=185} ("位置 2")) -> ("Top"=w378:i32)
              n174 = in-place-cluster #29(T6 {"Left"=674, "Top"=149} ("位置")) -> ("Top"=w379:i32)
              n175 = in-place-cluster #30(T6 {"Left"=674, "Top"=221} ("位置 3")) -> ("Top"=w371:i32)
              n176 = in-place-cluster #31(T6 {"Left"=674, "Top"=292} ("位置 5")) -> ("Top"=w376:i32)
              n177 = Subtract(x=w377, y=w372) -> (x-y=w373:i32)
              n178 = in-place-cluster #25("Top"=w373) -> (w350:T6)
              n179 = in-place-cluster #26("Top"=w375) -> (w359:T6)
              n180 = in-place-cluster #27("Top"=w374) -> (w361:T6)
              n181 = in-place-cluster #28("Top"=w378) -> (w354:T6)
              n182 = in-place-cluster #29("Top"=w379) -> (w356:T6)
              n183 = in-place-cluster #30("Top"=w371) -> (w352:T6)
              n184 = in-place-cluster #31("Top"=w376) -> (w358:T6)
            }
          }
          frame 4 {
            n185 = Unbundle By Name(w403) -> ("叶绿素a"=w402:u32)
            n186 = case shown="\"纳清\"" w420 {
              tunnel: [FALSE TRUE FALSE] -> w423
              tunnel: [0 ("y") 0 ("y") 36 ("y")] -> w415
              tunnel: [_ _ TRUE] -> w404
              tunnel: [_ _ string[] ["（0-500）μg/L", "（0-50）μg/L"]] -> w401
              tunnel: [_ _ w447] -> w400
              tunnel: [_ _ w446] -> w399
              tunnel: [_ _ w445] -> w398
              tunnel: [_ _ w444] -> w397
              tunnel: [_ _ TRUE] -> w396
              tunnel: [_ _ TRUE] -> w395
              tunnel: [_ _ TRUE] -> w394
              tunnel: [_ _ TRUE] -> w393
              frame "禹山", Default {
              }
              frame "国弘" {
              }
              frame "纳清" {
                n187 = global read "纳清过程全局变量.vi" "叶绿素a测试值"() -> (w448:T14)
                n188 = Unbundle By Name(w448) -> ("量程"=w447:u16, "清扫模式"=w446:u16, "清扫次数"=w445:u16, "清扫间隔分钟"=w444:u16)
              }
            }
            n189 = in-place {
              in-place-border: w415 -> [w427]
              n190 = in-place-cluster #32(T6 {"Left"=674, "Top"=256} ("位置 4")) -> ("Top"=w433:i32)
              n191 = in-place-cluster #33(T6 {"Left"=638, "Top"=366} ("位置 7")) -> ("Top"=w430:i32)
              n192 = in-place-cluster #34(T6 {"Left"=710, "Top"=328} ("位置 6")) -> ("Top"=w429:i32)
              n193 = in-place-cluster #35(T6 {"Left"=656, "Top"=185} ("位置 2")) -> ("Top"=w434:i32)
              n194 = in-place-cluster #36(T6 {"Left"=674, "Top"=149} ("位置")) -> ("Top"=w435:i32)
              n195 = in-place-cluster #37(T6 {"Left"=674, "Top"=221} ("位置 3")) -> ("Top"=w432:i32)
              n196 = in-place-cluster #38(T6 {"Left"=674, "Top"=292} ("位置 5")) -> ("Top"=w431:i32)
              n197 = Subtract(x=w432, y=w427) -> (x-y=w428:i32)
              n198 = in-place-cluster #32("Top"=w433) -> (w405:T6)
              n199 = in-place-cluster #33("Top"=w430) -> (w414:T6)
              n200 = in-place-cluster #34("Top"=w429) -> (w416:T6)
              n201 = in-place-cluster #35("Top"=w434) -> (w409:T6)
              n202 = in-place-cluster #36("Top"=w435) -> (w411:T6)
              n203 = in-place-cluster #37("Top"=w428) -> (w407:T6)
              n204 = in-place-cluster #38("Top"=w431) -> (w413:T6)
            }
          }
          frame 5 {
            n205 = Unbundle By Name(w463) -> ("藻密度"=w462:u32)
            n206 = case shown="\"纳清\"" w480 {
              tunnel: [FALSE TRUE FALSE] -> w483
              tunnel: [0 ("y") 0 ("y") 36 ("y")] -> w475
              tunnel: [_ _ TRUE] -> w464
              tunnel: [_ _ string[] ["（0-2000000）c/mL", "（0-200000）c/mL"]] -> w461
              tunnel: [_ _ w507] -> w460
              tunnel: [_ _ TRUE] -> w459
              tunnel: [_ _ w505] -> w458
              tunnel: [_ _ w504] -> w457
              tunnel: [_ _ w503] -> w456
              tunnel: [_ _ TRUE] -> w455
              tunnel: [_ _ TRUE] -> w454
              tunnel: [_ _ TRUE] -> w453
              frame "禹山", Default {
              }
              frame "国弘" {
              }
              frame "纳清" {
                n207 = global read "纳清过程全局变量.vi" "蓝绿藻测试值"() -> (w508:T15)
                n208 = Unbundle By Name(w508) -> ("量程"=w507:u16, "清扫模式"=w505:u16, "清扫次数"=w504:u16, "清扫间隔分钟"=w503:u16)
              }
            }
            n209 = in-place {
              in-place-border: w475 -> [w487]
              n210 = in-place-cluster #39(T6 {"Left"=674, "Top"=256} ("位置 4")) -> ("Top"=w493:i32)
              n211 = in-place-cluster #40(T6 {"Left"=638, "Top"=366} ("位置 7")) -> ("Top"=w490:i32)
              n212 = in-place-cluster #41(T6 {"Left"=710, "Top"=328} ("位置 6")) -> ("Top"=w489:i32)
              n213 = in-place-cluster #42(T6 {"Left"=656, "Top"=185} ("位置 2")) -> ("Top"=w494:i32)
              n214 = in-place-cluster #43(T6 {"Left"=674, "Top"=149} ("位置")) -> ("Top"=w495:i32)
              n215 = in-place-cluster #44(T6 {"Left"=674, "Top"=221} ("位置 3")) -> ("Top"=w492:i32)
              n216 = in-place-cluster #45(T6 {"Left"=674, "Top"=292} ("位置 5")) -> ("Top"=w491:i32)
              n217 = Subtract(x=w492, y=w487) -> (x-y=w488:i32)
              n218 = in-place-cluster #39("Top"=w493) -> (w465:T6)
              n219 = in-place-cluster #40("Top"=w490) -> (w474:T6)
              n220 = in-place-cluster #41("Top"=w489) -> (w476:T6)
              n221 = in-place-cluster #42("Top"=w494) -> (w469:T6)
              n222 = in-place-cluster #43("Top"=w495) -> (w471:T6)
              n223 = in-place-cluster #44("Top"=w488) -> (w467:T6)
              n224 = in-place-cluster #45("Top"=w491) -> (w473:T6)
            }
          }
          frame 6 {
            n225 = Unbundle By Name(w514) -> ("ORP"=w513:u32)
            n226 = case shown="\"国弘\"" w531 {
              tunnel: [FALSE TRUE] -> w534
              tunnel: [_ w549] -> w516
              tunnel: [w546 w548] -> w515
              tunnel: w513 -> [w546 _]
              frame "禹山", Default {
              }
              frame "国弘" {
                n227 = global read "国弘过程全局变量.vi" "ORP"() -> (w550:T16)
                n228 = Unbundle By Name(w550) -> ("命令滤波设定"=w548:u16, "偏移修正值"=w549:sgl)
              }
            }
            n229 = in-place {
              n230 = in-place-cluster #46(T6 {"Left"=674, "Top"=256} ("位置 4")) -> ("Top"=w543:i32)
              n231 = in-place-cluster #47(T6 {"Left"=638, "Top"=366} ("位置 7")) -> ("Top"=w539:i32)
              n232 = in-place-cluster #48(T6 {"Left"=710, "Top"=328} ("位置 6")) -> ("Top"=w540:i32)
              n233 = in-place-cluster #49(T6 {"Left"=656, "Top"=185} ("位置 2")) -> ("Top"=w544:i32)
              n234 = in-place-cluster #50(T6 {"Left"=674, "Top"=149} ("位置")) -> ("Top"=w545:i32)
              n235 = in-place-cluster #51(T6 {"Left"=674, "Top"=221} ("位置 3")) -> ("Top"=w542:i32)
              n236 = in-place-cluster #52(T6 {"Left"=674, "Top"=292} ("位置 5")) -> ("Top"=w541:i32)
              n237 = in-place-cluster #46("Top"=w543) -> (w517:T6)
              n238 = in-place-cluster #47("Top"=w539) -> (w526:T6)
              n239 = in-place-cluster #48("Top"=w540) -> (w527:T6)
              n240 = in-place-cluster #49("Top"=w544) -> (w521:T6)
              n241 = in-place-cluster #50("Top"=w545) -> (w523:T6)
              n242 = in-place-cluster #51("Top"=w542) -> (w519:T6)
              n243 = in-place-cluster #52("Top"=w541) -> (w525:T6)
            }
          }
          frame 7 {
            n244 = in-place {
              n245 = in-place-cluster #53(T6 {"Left"=674, "Top"=256} ("位置 4")) -> ("Top"=w580:i32)
              n246 = in-place-cluster #54(T6 {"Left"=638, "Top"=366} ("位置 7")) -> ("Top"=w576:i32)
              n247 = in-place-cluster #55(T6 {"Left"=710, "Top"=328} ("位置 6")) -> ("Top"=w577:i32)
              n248 = in-place-cluster #56(T6 {"Left"=656, "Top"=185} ("位置 2")) -> ("Top"=w581:i32)
              n249 = in-place-cluster #57(T6 {"Left"=674, "Top"=149} ("位置")) -> ("Top"=w582:i32)
              n250 = in-place-cluster #58(T6 {"Left"=674, "Top"=221} ("位置 3")) -> ("Top"=w579:i32)
              n251 = in-place-cluster #59(T6 {"Left"=674, "Top"=292} ("位置 5")) -> ("Top"=w578:i32)
              n252 = in-place-cluster #53("Top"=w580) -> (w555:T6)
              n253 = in-place-cluster #54("Top"=w576) -> (w564:T6)
              n254 = in-place-cluster #55("Top"=w577) -> (w565:T6)
              n255 = in-place-cluster #56("Top"=w581) -> (w559:T6)
              n256 = in-place-cluster #57("Top"=w582) -> (w561:T6)
              n257 = in-place-cluster #58("Top"=w579) -> (w557:T6)
              n258 = in-place-cluster #59("Top"=w578) -> (w563:T6)
            }
            n259 = global read "国弘过程全局变量.vi" "COD"() -> (w552:T17)
            n260 = Unbundle By Name(w552) -> ("数字滤波设定"=w554:u16, "COD偏移修正值"=w553:sgl)
          }
          frame 8 {
            n261 = Unbundle By Name(w587) -> ("DO"=w586:u32)
            n262 = case shown="\"禹山\", Default" w603 {
              tunnel: [FALSE TRUE] -> w606
              tunnel: [108 ("y") 72 ("y")] -> w598
              frame "禹山", Default {
              }
              frame "国弘" {
              }
            }
            n263 = in-place {
              in-place-border: w598 -> [w615]
              n264 = in-place-cluster #60(T6 {"Left"=674, "Top"=256} ("位置 4")) -> ("Top"=w612:i32)
              n265 = in-place-cluster #61(T6 {"Left"=638, "Top"=366} ("位置 7")) -> ("Top"=w619:i32)
              n266 = in-place-cluster #62(T6 {"Left"=710, "Top"=328} ("位置 6")) -> ("Top"=w621:i32)
              n267 = in-place-cluster #63(T6 {"Left"=656, "Top"=185} ("位置 2")) -> ("Top"=w613:i32)
              n268 = in-place-cluster #64(T6 {"Left"=674, "Top"=149} ("位置")) -> ("Top"=w614:i32)
              n269 = in-place-cluster #65(T6 {"Left"=674, "Top"=221} ("位置 3")) -> ("Top"=w611:i32)
              n270 = in-place-cluster #66(T6 {"Left"=674, "Top"=292} ("位置 5")) -> ("Top"=w617:i32)
              n271 = Subtract(x=w619, y=w615) -> (x-y=w618:i32)
              n272 = Subtract(x=w621, y=w615) -> (x-y=w620:i32)
              n273 = Subtract(x=w617, y=w615) -> (x-y=w616:i32)
              n274 = in-place-cluster #60("Top"=w612) -> (w588:T6)
              n275 = in-place-cluster #61("Top"=w618) -> (w597:T6)
              n276 = in-place-cluster #62("Top"=w620) -> (w599:T6)
              n277 = in-place-cluster #63("Top"=w613) -> (w592:T6)
              n278 = in-place-cluster #64("Top"=w614) -> (w594:T6)
              n279 = in-place-cluster #65("Top"=w611) -> (w590:T6)
              n280 = in-place-cluster #66("Top"=w616) -> (w596:T6)
            }
            n281 = global read "禹山过程全局变量.vi" "DO 2"() -> (w585:cluster{"温度测量值":sgl, "DO%":sgl, "DOmg/L":sgl})
            n282 = Unbundle By Name(w585) -> ("DOmg/L"=w584:sgl)
          }
          frame 9 {
            n283 = in-place {
              n284 = in-place-cluster #67(T6 {"Left"=674, "Top"=256} ("位置 4")) -> ("Top"=w654:i32)
              n285 = in-place-cluster #68(T6 {"Left"=638, "Top"=366} ("位置 7")) -> ("Top"=w650:i32)
              n286 = in-place-cluster #69(T6 {"Left"=710, "Top"=328} ("位置 6")) -> ("Top"=w651:i32)
              n287 = in-place-cluster #70(T6 {"Left"=656, "Top"=185} ("位置 2")) -> ("Top"=w655:i32)
              n288 = in-place-cluster #71(T6 {"Left"=674, "Top"=149} ("位置")) -> ("Top"=w656:i32)
              n289 = in-place-cluster #72(T6 {"Left"=674, "Top"=221} ("位置 3")) -> ("Top"=w653:i32)
              n290 = in-place-cluster #73(T6 {"Left"=674, "Top"=292} ("位置 5")) -> ("Top"=w652:i32)
              n291 = in-place-cluster #67("Top"=w654) -> (w629:T6)
              n292 = in-place-cluster #68("Top"=w650) -> (w638:T6)
              n293 = in-place-cluster #69("Top"=w651) -> (w639:T6)
              n294 = in-place-cluster #70("Top"=w655) -> (w633:T6)
              n295 = in-place-cluster #71("Top"=w656) -> (w635:T6)
              n296 = in-place-cluster #72("Top"=w653) -> (w631:T6)
              n297 = in-place-cluster #73("Top"=w652) -> (w637:T6)
            }
            n298 = global read "国弘过程全局变量.vi" "氯化物"() -> (w626:T18)
            n299 = Unbundle By Name(w626) -> ("命令滤波设定"=w628:u16, "偏移修正值"=w627:sgl)
          }
          frame 10 {
            n300 = Unbundle By Name(w657) -> ("氨氮"=w658:u32)
            n301 = in-place {
              n302 = in-place-cluster #74(T6 {"Left"=674, "Top"=256} ("位置 4")) -> ("Top"=w684:i32)
              n303 = in-place-cluster #75(T6 {"Left"=638, "Top"=366} ("位置 7")) -> ("Top"=w680:i32)
              n304 = in-place-cluster #76(T6 {"Left"=710, "Top"=328} ("位置 6")) -> ("Top"=w681:i32)
              n305 = in-place-cluster #77(T6 {"Left"=656, "Top"=185} ("位置 2")) -> ("Top"=w685:i32)
              n306 = in-place-cluster #78(T6 {"Left"=674, "Top"=149} ("位置")) -> ("Top"=w686:i32)
              n307 = in-place-cluster #79(T6 {"Left"=674, "Top"=221} ("位置 3")) -> ("Top"=w683:i32)
              n308 = in-place-cluster #80(T6 {"Left"=674, "Top"=292} ("位置 5")) -> ("Top"=w682:i32)
              n309 = in-place-cluster #74("Top"=w684) -> (w659:T6)
              n310 = in-place-cluster #75("Top"=w680) -> (w668:T6)
              n311 = in-place-cluster #76("Top"=w681) -> (w669:T6)
              n312 = in-place-cluster #77("Top"=w685) -> (w663:T6)
              n313 = in-place-cluster #78("Top"=w686) -> (w665:T6)
              n314 = in-place-cluster #79("Top"=w683) -> (w661:T6)
              n315 = in-place-cluster #80("Top"=w682) -> (w667:T6)
            }
          }
          frame 11 {
            n316 = global read "国弘过程全局变量.vi" "水中油"() -> (w687:T19)
            n317 = Unbundle By Name(w687) -> ("数位滤波设定"=w691:u16, "水中油B值"=w692:sgl, "清洁周期"=w690:u16)
            n318 = in-place {
              in-place-border: 0 ("y") -> [w714]
              n319 = in-place-cluster #81(T6 {"Left"=674, "Top"=256} ("位置 4")) -> ("Top"=w720:i32)
              n320 = in-place-cluster #82(T6 {"Left"=638, "Top"=366} ("位置 7")) -> ("Top"=w717:i32)
              n321 = in-place-cluster #83(T6 {"Left"=710, "Top"=328} ("位置 6")) -> ("Top"=w716:i32)
              n322 = in-place-cluster #84(T6 {"Left"=656, "Top"=185} ("位置 2")) -> ("Top"=w721:i32)
              n323 = in-place-cluster #85(T6 {"Left"=674, "Top"=149} ("位置")) -> ("Top"=w722:i32)
              n324 = in-place-cluster #86(T6 {"Left"=674, "Top"=221} ("位置 3")) -> ("Top"=w719:i32)
              n325 = in-place-cluster #87(T6 {"Left"=674, "Top"=292} ("位置 5")) -> ("Top"=w718:i32)
              n326 = Subtract(x=w719, y=w714) -> (x-y=w715:i32)
              n327 = in-place-cluster #81("Top"=w720) -> (w693:T6)
              n328 = in-place-cluster #82("Top"=w717) -> (w702:T6)
              n329 = in-place-cluster #83("Top"=w716) -> (w704:T6)
              n330 = in-place-cluster #84("Top"=w721) -> (w697:T6)
              n331 = in-place-cluster #85("Top"=w722) -> (w699:T6)
              n332 = in-place-cluster #86("Top"=w715) -> (w695:T6)
              n333 = in-place-cluster #87("Top"=w718) -> (w701:T6)
            }
          }
        }
        n334 = property on="BT" class="DigNum (strict)"("Visible"=w128) -> ()  [unwired: 2 in, 2 out]
        n335 = property on="KT" class="DigNum (strict)"("Visible"=w128) -> ()  [unwired: 2 in, 2 out]
        n336 = property on="恢复出厂" class="Bool"("Visible"=w130) -> ()  [unwired: 2 in, 2 out]
        n337 = property on="温度校准系数读取" class="Bool"("Visible"=w128) -> ()  [unwired: 2 in, 2 out]
        n338 = property on="温度校准系数写入" class="Bool"("Visible"=w128) -> ()  [unwired: 2 in, 2 out]
        n339 = property on="校准温度" class="Bool"("DisabledEnum"=w129) -> ()  [unwired: 2 in, 2 out]
        n340 = global read "断电保存变量.vi" "大气压补偿"() -> (w147:dbl)
        n341 = global read "断电保存变量.vi" "盐度自动获取"() -> (w146:bool)
        n342 = property on="温度系数" class="DigNum (strict)"("Position"=w158, "Visible"=w151) -> ()  [unwired: 2 in, 2 out]
        n343 = property on="清扫次数" class="DigNum (strict)"("Visible"=w138, "Value"=w136) -> ()  [unwired: 2 in, 2 out]
        n344 = property on="清洗选板" class="TabCtl (strict)"("Visible"=w134) -> ()  [unwired: 2 in, 2 out]
        n345 = property on="盐度" class="DigNum (strict)"("Position"=w156, "Visible"=w152) -> ()  [unwired: 2 in, 2 out]
        n346 = property on="滤波次数" class="DigNum (strict)"("Position"=w162, "Visible"=w154, "Value"=w145) -> ()  [unwired: 2 in, 2 out]
        n347 = property on="清扫间隔" class="DigNum (strict)"("Visible"=w139, "Value"=w140) -> ()  [unwired: 2 in, 2 out]
        n348 = property on="测量量程" class="Ring (strict)"("Position"=w159, "Visible"=w153, "Strings []"=w142, "Value"=w141) -> ()  [unwired: 2 in, 2 out]
        n349 = property on="清扫模式" class="Ring (strict)"("Visible"=w137, "Value"=w135) -> ()  [unwired: 2 in, 2 out]
        n350 = property on="大气压力" class="DigNum (strict)"("Position"=w157, "Visible"=w148, "Value"=w147) -> ()  [unwired: 2 in, 2 out]
        n351 = property on="溶解氧浓度值" class="DigNum (strict)"("Visible"=w133, "Value"=w132) -> ()  [unwired: 2 in, 2 out]
        n352 = property on="自动盐度补偿" class="Bool (strict)"("Position"=w155, "Visible"=w149, "Value"=w146) -> ()  [unwired: 2 in, 2 out]
        n353 = property on="偏移修正值" class="DigNum (strict)"("Position"=w160, "Visible"=w150, "Value"=w144) -> ()  [unwired: 2 in, 2 out]
      }
    }
  }
  n354 = while {
    tunnel: w1 -> [w723]
    stop <- FALSE stop-if-true
    n355 = event shown="[5] \"恢复出厂\": Value Change" {
      selector: _ -> [_ _ _ _ _ _ _ _ _ _ _ _ _ _ _ _ _ _ _ _ _]
      dyn-events: _ -> [_ _ _ _ _ _ _ _ _ _ _ _ _ _ _ _ _ _ _ _ _]
      timeout: _ -> [_ _ _ _ _ _ _ _ _ _ _ _ _ _ _ _ _ _ _ _ _]
      tunnel: w723 -> [_ _ _ w761 _ _ _ _ _ _ _ _ _ _ _ _ _ _ _ _ _]
      event Timeout {
        n356 = event-data() -> ()  [unwired: 1 in, 3 out]
      }
      event "温度校准系数读取": Value Change {
        n357 = event-data() -> ()  [unwired: 1 in, 6 out]
        n358 = local read "校准参数"() -> (w725:u16)
        n359 = case shown="6" w725 {
          tunnel: [T20."null" ("探头") T20."pH" ("探头") T20."DO" ("探头") T20."浊度" ("探头") T20."电导率" ("探头") T20."叶绿素a" ("探头") T20."DO2" ("探头") T20."藻密度" ("探头")] -> w726
          frame Default {
          }
          frame 0 {
          }
          frame 1 {
          }
          frame 2 {
          }
          frame 3 {
          }
          frame 4 {
          }
          frame 5 {
          }
          frame 6 {
          }
        }
        n360 = global read "多参数全局变量.vi" "MB session in"() -> (w727:refnum<class "MB_Master.lvclass">)
        n361 = call "STD获取温度校准参数.vi"("探头"=w726, "MB session in"=w727) -> ("error out"=w728:errorcluster, "输出值"=w732:cluster{"K":sgl, "B":sgl})  [unwired: 7 in, 1 out]
        n362 = case shown="No Error" w728 {
          tunnel: ["读取成功！" "读取失败！"] -> w729
          frame No Error {
          }
          frame Error {
          }
        }
        n363 = Unbundle By Name(w732) -> ("K"=w731:sgl, "B"=w730:sgl)
        n364 = local write "KT"(w731) -> ()
        n365 = local write "BT"(w730) -> ()
        n366 = One Button Dialog(message=w729) -> ()  [unwired: 1 in, 1 out]
      }
      event "温度校准系数写入": Value Change {
        n367 = event-data() -> ()  [unwired: 1 in, 6 out]
        n368 = local read "校准参数"() -> (w745:u16)
        n369 = case shown="6" w745 {
          tunnel: [T20."null" ("探头") T20."pH" ("探头") T20."DO" ("探头") T20."浊度" ("探头") T20."电导率" ("探头") T20."叶绿素a" ("探头") T20."DO2" ("探头") T20."藻密度" ("探头")] -> w746
          frame Default {
          }
          frame 0 {
          }
          frame 1 {
          }
          frame 2 {
          }
          frame 3 {
          }
          frame 4 {
          }
          frame 5 {
          }
          frame 6 {
          }
        }
        n370 = global read "多参数全局变量.vi" "MB session in"() -> (w747:refnum<class "MB_Master.lvclass">)
        n371 = Bundle("KT"="KT", "BT"="BT") -> (w748:cluster{"KT":dbl, "BT":dbl})  [unwired: 1 in]
        n372 = call "STD设置温度校准参数.vi"("探头"=w746, "用户校准参数"=w748, "MB session in"=w747) -> ("error out"=w744:errorcluster)  [unwired: 7 in, 1 out]
        n373 = case shown="Error" w744 {
          tunnel: ["写入成功！" "写入失败！"] -> w743
          frame No Error {
          }
          frame Error {
          }
        }
        n374 = One Button Dialog(message=w743) -> ()  [unwired: 1 in, 1 out]
      }
      event "显示曲线": Value Change {
        n375 = event-data() -> ()  [unwired: 1 in, 6 out]
        n376 = Set Occurrence(w761) -> ()
      }
      event "温度系数": Value Change {
        n377 = event-data() -> ()  [unwired: 1 in, 6 out]
        n378 = property on="校准参数" class="Ring (strict)"() -> ("Value"=w765:u16)  [unwired: 2 in, 2 out]
        n379 = call "探头温度系数.vi"("校准参数"=w765, "温度系数"="温度系数") -> ("error out"=w762:errorcluster)  [unwired: 9 in]
        n380 = case shown="Error" w762 {
          tunnel: ["设置成功！" "设置失败！"] -> w763
          frame No Error {
          }
          frame Error {
          }
        }
        n381 = One Button Dialog(message=w763) -> ()  [unwired: 1 in, 1 out]
      }
      event "恢复出厂": Value Change {
        n382 = event-data() -> ()  [unwired: 1 in, 6 out]
        n383 = property on="校准参数" class="Ring (strict)"() -> ("Value"=w770:u16)  [unwired: 2 in, 2 out]
        n384 = call "探头恢复出厂.vi"("校准参数"=w770) -> ("error out"=w768:errorcluster)  [unwired: 10 in]
        n385 = case shown="Error" w768 {
          tunnel: ["设置成功！" "设置失败！"] -> w769
          frame No Error {
          }
          frame Error {
          }
        }
        n386 = One Button Dialog(message=w769) -> ()  [unwired: 1 in, 1 out]
      }
      event "测量量程": Value Change {
        n387 = event-data() -> ()  [unwired: 1 in, 6 out]
        n388 = property on="校准参数" class="Ring (strict)"() -> ("Value"=w775:u16)  [unwired: 2 in, 2 out]
        n389 = call "探头校准量程设置.vi"("校准参数"=w775, "校准量程"="测量量程") -> ("error out"=w774:errorcluster)  [unwired: 9 in]
        n390 = call "探头测量量程设置.vi"("校准参数"=w775, "error in (no error)"=w774, "测量量程设置"="测量量程") -> ("error out"=w776:errorcluster)  [unwired: 8 in]
        n391 = case shown="Error" w776 {
          tunnel: ["设置成功！" "设置失败！"] -> w777
          frame No Error {
          }
          frame Error {
          }
        }
        n392 = One Button Dialog(message=w777) -> ()  [unwired: 1 in, 1 out]
      }
      event "自动盐度补偿", "大气压力", "盐度", "滤波次数": Value Change {
        n393 = event-data() -> ()  [unwired: 1 in, 6 out]
        n394 = flat-sequence {
          tunnel: [w781] -> w780
          tunnel: w780 -> [_]
          frame #0 {
            n395 = property on="校准参数" class="Ring (strict)"() -> ("Value"=w783:u16)  [unwired: 2 in, 2 out]
            n396 = global write "断电保存变量.vi" "盐度补偿"("盐度") -> ()
            n397 = global write "断电保存变量.vi" "大气压补偿"("大气压力") -> ()
            n398 = call "探头滤波次数.vi"("校准参数"=w783, "滤波次数"="滤波次数") -> ("error out"=w781:errorcluster)  [unwired: 9 in]
            n399 = global write "断电保存变量.vi" "盐度自动获取"("自动盐度补偿") -> ()
          }
          frame #1 {
            n400 = call "配置文件保存.vi"() -> ()  [unwired: 12 in]
          }
        }
      }
      event "清洗": Value Change {
        n401 = event-data() -> ()  [unwired: 1 in, 6 out]
        n402 = property on="校准参数" class="Ring (strict)"() -> ("Value"=w787:u16)  [unwired: 2 in, 2 out]
        n403 = call "探头手动清洗.vi"("校准参数"=w787) -> ("error out"=w788:errorcluster)  [unwired: 10 in]
        n404 = case shown="No Error" w788 {
          tunnel: ["启动成功！" "启动失败！"] -> w789
          frame No Error {
          }
          frame Error {
          }
        }
        n405 = One Button Dialog(message=w789) -> ()  [unwired: 1 in, 1 out]
      }
      event "清扫模式": Value Change {
        n406 = event-data() -> ()  [unwired: 1 in, 6 out]
        n407 = property on="校准参数" class="Ring (strict)"() -> ("Value"=w793:u16)  [unwired: 2 in, 2 out]
        n408 = case shown="5" w793 {
          tunnel: [T21."null" ("探头") T21."pH" ("探头") T21."DO" ("探头") T21."浊度" ("探头") T21."电导率" ("探头") T21."叶绿素a" ("探头") T21."藻密度" ("探头") 17] -> w792
          frame Default {
          }
          frame 0 {
          }
          frame 1 {
          }
          frame 2 {
          }
          frame 3 {
          }
          frame 4 {
          }
          frame 5 {
          }
          frame 11 {
          }
        }
        n409 = call "纳清_清扫模式.vi"("探头"=w792, "清扫模式"="清扫模式") -> ("error out"=w794:errorcluster)  [unwired: 9 in]
        n410 = case shown="Error" w794 {
          tunnel: ["设置成功！" "设置失败！"] -> w795
          frame No Error {
          }
          frame Error {
          }
        }
        n411 = One Button Dialog(message=w795) -> ()  [unwired: 1 in, 1 out]
      }
      event "清扫次数": Value Change {
        n412 = event-data() -> ()  [unwired: 1 in, 6 out]
        n413 = property on="校准参数" class="Ring (strict)"() -> ("Value"=w811:u16)  [unwired: 2 in, 2 out]
        n414 = case shown="11" w811 {
          tunnel: [T21."null" ("探头") T21."pH" ("探头") T21."DO" ("探头") T21."浊度" ("探头") T21."电导率" ("探头") T21."叶绿素a" ("探头") T21."藻密度" ("探头") 17] -> w810
          frame Default {
          }
          frame 0 {
          }
          frame 1 {
          }
          frame 2 {
          }
          frame 3 {
          }
          frame 4 {
          }
          frame 5 {
          }
          frame 11 {
          }
        }
        n415 = call "纳清_清扫次数.vi"("探头"=w810, "清扫次数"="清扫次数") -> ("error out"=w808:errorcluster)  [unwired: 9 in]
        n416 = case shown="Error" w808 {
          tunnel: ["设置成功！" "设置失败！"] -> w809
          frame No Error {
          }
          frame Error {
          }
        }
        n417 = One Button Dialog(message=w809) -> ()  [unwired: 1 in, 1 out]
      }
      event "清扫间隔": Value Change {
        n418 = event-data() -> ()  [unwired: 1 in, 6 out]
        n419 = property on="校准参数" class="Ring (strict)"() -> ("Value"=w823:u16)  [unwired: 2 in, 2 out]
        n420 = call "探头清洗间隔.vi"("校准参数"=w823, "清扫间隔"="清扫间隔") -> ("error out"=w822:errorcluster)  [unwired: 9 in]
        n421 = case shown="Error" w822 {
          tunnel: ["设置成功！" "设置失败！"] -> w825
          frame No Error {
          }
          frame Error {
          }
        }
        n422 = One Button Dialog(message=w825) -> ()  [unwired: 1 in, 1 out]
      }
      event "校准温度": Value Change {
        n423 = event-data() -> ()  [unwired: 1 in, 6 out]
        n424 = property on="校准参数" class="Ring (strict)"() -> ("Value"=w831:u16)  [unwired: 2 in, 2 out]
        n425 = call "温度校准.vi"("校准参数"=w831, "校准温度"="实际温度") -> ("error out"=w830:errorcluster)  [unwired: 9 in]
        n426 = case shown="Error" w830 {
          tunnel: ["校准成功！" "校准失败！"] -> w829
          frame No Error {
          }
          frame Error {
          }
        }
        n427 = One Button Dialog(message=w829) -> ()  [unwired: 1 in, 1 out]
      }
      event "偏移修正值": Value Change {
        n428 = event-data() -> ()  [unwired: 1 in, 6 out]
        n429 = property on="校准参数" class="Ring (strict)"() -> ("Value"=w835:u16)  [unwired: 2 in, 2 out]
        n430 = call "探头偏移修正值.vi"("校准参数"=w835, "温度偏移修正值"="偏移修正值") -> ("error out"=w836:errorcluster)  [unwired: 9 in]
        n431 = case shown="No Error" w836 {
          tunnel: ["设置成功！" "设置失败！"] -> w837
          frame No Error {
          }
          frame Error {
          }
        }
        n432 = One Button Dialog(message=w837) -> ()  [unwired: 1 in, 1 out]
      }
      event "标液一.标准值", "标液二.标准值", "标液三.标准值", "实际温度", "大气压力", "盐度", "滤波次数", "偏移修正值", "温度系数", "标液一.原始值", "标液三.原始值", "标液二.原始值": Mouse Down {
        n433 = event-data() -> ("CtlRef"=w843:refnum<vi>)  [unwired: 1 in, 7 out]
        n434 = property class="DigNum (strict)"(reference=w843) -> (reference out=w841:refnum<vi>, "Value"=w842:dbl)  [unwired: 1 in, 1 out]
        n435 = call "数字键盘.vi"("OldNumber"=w842) -> ("NewNumber"=w840:dbl)  [unwired: 1 in]
        n436 = property class="DigNum (strict)"(reference=w841, "Val(Sgnl)"=w840) -> ()  [unwired: 1 in, 2 out]
      }
      event "清扫次数", "清扫间隔": Mouse Down {
        n437 = event-data() -> ("CtlRef"=w847:refnum<vi>)  [unwired: 1 in, 7 out]
        n438 = property class="DigNum (strict)"(reference=w847) -> (reference out=w845:refnum<vi>, "Value"=w846:u16)  [unwired: 1 in, 1 out]
        n439 = call "数字键盘.vi"("OldNumber"=w846) -> ("NewNumber"=w844:dbl)  [unwired: 1 in]
        n440 = property class="DigNum (strict)"(reference=w845, "Val(Sgnl)"=w844) -> ()  [unwired: 1 in, 2 out]
      }
      event "标液一.标准值", "标液二.标准值", "标液三.标准值": Value Change {
        n441 = event-data() -> ()  [unwired: 1 in, 6 out]
        n442 = property on="校准参数" class="Ring (strict)"() -> ("Value"=w851:u16)  [unwired: 2 in, 2 out]
        n443 = property on="标准值" class="DigNum (strict)"() -> ("Value"=w850:dbl)  [unwired: 2 in, 2 out]
        n444 = property on="标准值" class="DigNum (strict)"() -> ("Value"=w849:dbl)  [unwired: 2 in, 2 out]
        n445 = property on="标准值" class="DigNum (strict)"() -> ("Value"=w848:dbl)  [unwired: 2 in, 2 out]
        n446 = call "探头校准标准值设置.vi"("校准参数"=w851, "标液三"=w848, "标液二"=w849, "标液一"=w850) -> ()  [unwired: 8 in]
      }
      event "校准参数": Value Change {
        n447 = event-data() -> ()  [unwired: 1 in, 6 out]
        n448 = property on="校准参数" class="Ring (strict)"() -> ("Value"=w854:u16)  [unwired: 2 in, 2 out]
        n449 = call "探头型号.vi"("校准参数"=w854) -> ("禁用项[]"=w853:i32[], "value"=w852:i32)  [unwired: 8 in, 1 out]
        n450 = property on="校准方式" class="Ring (strict)"("Disabled Items []"=w853, "Val(Sgnl)"=w852) -> ()  [unwired: 2 in, 2 out]
      }
      event "校准方式": Value Change {
        n451 = event-data() -> ()  [unwired: 1 in, 6 out]
        n452 = property on="校准参数" class="Ring (strict)"() -> ("Value"=w857:u16)  [unwired: 2 in, 2 out]
        n453 = call "探头型号.vi"("校准参数"=w857) -> ("探头型号"=w856:T3)  [unwired: 8 in, 2 out]
        n454 = case shown="\"禹山\", Default" w856 {
          tunnel: [_ TRUE] -> w855
          frame "禹山", Default {
          }
          frame "国弘" {
          }
        }
        n455 = flat-sequence {
          tunnel: w855 -> [w859]
          frame #0 {
            n456 = property on="校准方式" class="Ring (strict)"() -> ("Value"=w858:u16)  [unwired: 2 in, 2 out]
            n457 = case shown="2" w858 {
              tunnel: [cluster{bool, bool, bool} {TRUE, FALSE, FALSE} cluster{bool, bool, bool} {TRUE, TRUE, FALSE} cluster{bool, bool, bool} {TRUE, TRUE, TRUE}] -> w865
              frame 0, Default {
              }
              frame 1 {
              }
              frame 2 {
              }
            }
            n458 = Unbundle(w865) -> (w864:bool, w862:bool, w863:bool)
            n459 = property on="标液一" class="Clust (strict)"("Visible"=w864) -> ()  [unwired: 2 in, 2 out]
            n460 = property on="标液二" class="Clust (strict)"("Visible"=w862) -> ()  [unwired: 2 in, 2 out]
            n461 = property on="标液三" class="Clust (strict)"("Visible"=w863) -> ()  [unwired: 2 in, 2 out]
            n462 = And(x=w859, y=w862) -> (x .and. y?=w861:bool)
            n463 = And(x=w863, y=w859) -> (x .and. y?=w860:bool)
            n464 = property on="第一点确认校准" class="Bool"("Visible"=w864) -> ()  [unwired: 2 in, 2 out]
            n465 = property on="标液一开始校准" class="Bool (strict)"("Visible"=w864) -> ()  [unwired: 2 in, 2 out]
            n466 = property on="标液二开始校准" class="Bool (strict)"("Visible"=w862) -> ()  [unwired: 2 in, 2 out]
            n467 = property on="标液三开始校准" class="Bool (strict)"("Visible"=w863) -> ()  [unwired: 2 in, 2 out]
            n468 = property on="第二点确认校准" class="Bool"("Visible"=w861) -> ()  [unwired: 2 in, 2 out]
            n469 = property on="第三点确认校准" class="Bool"("Visible"=w860) -> ()  [unwired: 2 in, 2 out]
          }
        }
      }
      event "标液一开始校准", "标液二开始校准", "标液三开始校准": Value Change {
        n470 = event-data() -> ("CtlRef"=w882:refnum<vi>, "NewVal"=w870:bool)  [unwired: 1 in, 4 out]
        n471 = case shown="True" w870 {
          tunnel: [_ w884] -> w871
          frame False {
          }
          frame True {
            n472 = property on="校准参数" class="Ring (strict)"() -> ("Value"=w883:u16)  [unwired: 2 in, 2 out]
            n473 = case shown="7" w883 {
              tunnel: [T2 {"ph"=TRUE, "DO"=FALSE, "Cond"=FALSE, "Turb"=FALSE, "叶绿素a"=FALSE, "藻密度"=FALSE, "ORP"=FALSE, "COD"=FALSE, "DO2"=FALSE, FALSE, "氨氮"=FALSE, "水中油"=FALSE} ("校准运行状态") T2 {"ph"=FALSE, "DO"=TRUE, "Cond"=FALSE, "Turb"=FALSE, "叶绿素a"=FALSE, "藻密度"=FALSE, "ORP"=FALSE, "COD"=FALSE, "DO2"=FALSE, FALSE, "氨氮"=FALSE, "水中油"=FALSE} ("校准运行状态") T2 {"ph"=FALSE, "DO"=FALSE, "Cond"=FALSE, "Turb"=TRUE, "叶绿素a"=FALSE, "藻密度"=FALSE, "ORP"=FALSE, "COD"=FALSE, "DO2"=FALSE, FALSE, "氨氮"=FALSE, "水中油"=FALSE} ("校准运行状态") T2 {"ph"=FALSE, "DO"=FALSE, "Cond"=TRUE, "Turb"=FALSE, "叶绿素a"=FALSE, "藻密度"=FALSE, "ORP"=FALSE, "COD"=FALSE, "DO2"=FALSE, FALSE, "氨氮"=FALSE, "水中油"=FALSE} ("校准运行状态") T2 {"ph"=FALSE, "DO"=FALSE, "Cond"=FALSE, "Turb"=FALSE, "叶绿素a"=TRUE, "藻密度"=FALSE, "ORP"=FALSE, "COD"=FALSE, "DO2"=FALSE, FALSE, "氨氮"=FALSE, "水中油"=FALSE} ("校准运行状态") T2 {"ph"=FALSE, "DO"=FALSE, "Cond"=FALSE, "Turb"=FALSE, "叶绿素a"=FALSE, "藻密度"=TRUE, "ORP"=FALSE, "COD"=FALSE, "DO2"=FALSE, FALSE, "氨氮"=FALSE, "水中油"=FALSE} ("校准运行状态") T2 {"ph"=FALSE, "DO"=FALSE, "Cond"=FALSE, "Turb"=FALSE, "叶绿素a"=FALSE, "藻密度"=FALSE, "ORP"=TRUE, "COD"=FALSE, "DO2"=FALSE, FALSE, "氨氮"=FALSE, "水中油"=FALSE} ("校准运行状态") T2 {"ph"=FALSE, "DO"=FALSE, "Cond"=FALSE, "Turb"=FALSE, "叶绿素a"=FALSE, "藻密度"=FALSE, "ORP"=FALSE, "COD"=TRUE, "DO2"=FALSE, FALSE, "氨氮"=FALSE, "水中油"=FALSE} ("校准运行状态") T2 {"ph"=FALSE, "DO"=FALSE, "Cond"=FALSE, "Turb"=FALSE, "叶绿素a"=FALSE, "藻密度"=FALSE, "ORP"=FALSE, "COD"=FALSE, "DO2"=TRUE, FALSE, "氨氮"=FALSE, "水中油"=FALSE} ("校准运行状态") T2 {"ph"=FALSE, "DO"=FALSE, "Cond"=FALSE, "Turb"=FALSE, "叶绿素a"=FALSE, "藻密度"=FALSE, "ORP"=FALSE, "COD"=FALSE, "DO2"=FALSE, TRUE, "氨氮"=FALSE, "水中油"=FALSE} ("校准运行状态") T2 {"ph"=FALSE, "DO"=FALSE, "Cond"=FALSE, "Turb"=FALSE, "叶绿素a"=FALSE, "藻密度"=FALSE, "ORP"=FALSE, "COD"=FALSE, "DO2"=FALSE, FALSE, "氨氮"=TRUE, "水中油"=FALSE} ("校准运行状态") T2 {"ph"=FALSE, "DO"=FALSE, "Cond"=FALSE, "Turb"=FALSE, "叶绿素a"=FALSE, "藻密度"=FALSE, "ORP"=FALSE, "COD"=FALSE, "DO2"=FALSE, FALSE, "氨氮"=FALSE, "水中油"=TRUE} ("校准运行状态")] -> w884
              frame 0, Default {
              }
              frame 1 {
              }
              frame 2 {
              }
              frame 3 {
              }
              frame 4 {
              }
              frame 5 {
              }
              frame 6 {
              }
              frame 7 {
              }
              frame 8 {
              }
              frame 9 {
              }
              frame 10 {
              }
              frame 11 {
              }
            }
          }
        }
        n474 = property class="Bool (strict)"(reference=w882) -> ("Label.Text"=w881:string)  [unwired: 1 in, 2 out]
        n475 = case shown="\"标液三开始校准\"" w881 {
          tunnel: [w898 w900 w902] -> _
          tunnel: [T22 {"禁用"=enum."Enabled", "禁用 2"=enum."Disabled and Grayed Out", "禁用 3"=enum."Disabled and Grayed Out"} T22 {"禁用"=enum."Disabled and Grayed Out", "禁用 2"=enum."Enabled", "禁用 3"=enum."Disabled and Grayed Out"} T22 {"禁用"=enum."Disabled and Grayed Out", "禁用 2"=enum."Disabled and Grayed Out", "禁用 3"=enum."Enabled"}] -> w879
          frame "标液一开始校准", Default {
            w898 = u16 0 items=["第一点", "第二点", "第三点"] ("当前校准点位")
          }
          frame "标液二开始校准" {
            w900 = u16 1 items=["第一点", "第二点", "第三点"] ("当前校准点位")
          }
          frame "标液三开始校准" {
            w902 = u16 2 items=["第一点", "第二点", "第三点"] ("当前校准点位")
          }
        }
        n476 = Select(t=T5."Disabled and Grayed Out" ("禁用 3"), s=w870, f=T5."Enabled") -> (s? t:f=w872:T5)
        n477 = property on="校准参数" class="Ring (strict)"("DisabledEnum"=w872) -> ()  [unwired: 2 in, 2 out]
        n478 = property on="校准方式" class="Ring (strict)"("DisabledEnum"=w872) -> ()  [unwired: 2 in, 2 out]
        n479 = property on="第一点确认校准" class="Bool"("DisabledEnum"=w872) -> ()  [unwired: 2 in, 2 out]
        n480 = property on="第二点确认校准" class="Bool"("DisabledEnum"=w872) -> ()  [unwired: 2 in, 2 out]
        n481 = property on="第三点确认校准" class="Bool"("DisabledEnum"=w872) -> ()  [unwired: 2 in, 2 out]
        n482 = global write "多参数全局变量.vi" "校准运行状态"(w871) -> ()
        n483 = Select(t=w879, s=w870, f=T22 {"禁用"=enum."Enabled", "禁用 2"=enum."Enabled", "禁用 3"=enum."Enabled"}) -> (s? t:f=w878:T22)
        n484 = Unbundle(w878) -> ("禁用"=w880:T5, "禁用 2"=w874:T5, "禁用 3"=w873:T5)
        n485 = property on="标液一开始校准" class="Bool (strict)"("DisabledEnum"=w880) -> ()  [unwired: 2 in, 2 out]
        n486 = property on="标液二开始校准" class="Bool (strict)"("DisabledEnum"=w874) -> ()  [unwired: 2 in, 2 out]
        n487 = property on="标液三开始校准" class="Bool (strict)"("DisabledEnum"=w873) -> ()  [unwired: 2 in, 2 out]
      }
      event "第一点确认校准", "第二点确认校准", "第三点确认校准": Value Change {
        n488 = event-data() -> ("CtlRef"=w917:refnum<vi>)  [unwired: 1 in, 5 out]
        n489 = property on="校准参数" class="Ring (strict)"() -> ("Value"=w912:u16)  [unwired: 2 in, 2 out]
        n490 = call "探头型号.vi"("校准参数"=w912) -> ("探头型号"=w918:T3)  [unwired: 8 in, 2 out]
        n491 = property on="校准参数" class="Ring (strict)"() -> ("Value"=w910:u16)  [unwired: 2 in, 2 out]
        n492 = property on="校准方式" class="Ring (strict)"() -> ("Value"=w909:u16)  [unwired: 2 in, 2 out]
        n493 = case shown="\"禹山\", Default" w918 {
          tunnel: [w945 w957] -> w906
          tunnel: w917 -> [_ w960]
          tunnel: [TRUE w947] -> w911
          tunnel: w909 -> [_ w958]
          tunnel: w910 -> [_ _]
          tunnel: [errorcluster {"status"=FALSE, "code"=0, "source"="校准成功！"} ("error in (no error)") w949] -> w905
          tunnel: [errorcluster {"status"=TRUE, "code"=0, "source"="校准失败！"} ("error in (no error)") w948] -> w904
          frame "禹山", Default {
            n494 = property on="校准方式" class="Ring (strict)"() -> ("Value"=w945:u16)  [unwired: 2 in, 2 out]
          }
          frame "国弘" {
            n495 = property class="Bool"(reference=w960) -> ("Label.Text"=w959:string)  [unwired: 1 in, 2 out]
            n496 = case shown="\"第一点确认校准\", Default" w959 {
              tunnel: [u16 0 ("Value") u16 1 ("Value") u16 2 ("Value")] -> w957
              tunnel: ["第一点校准通过，请更换标液，准备第二点校准！" "第二点校准通过，请更换标液，准备第三点校准！" "校准成功！"] -> w956
              tunnel: ["第一点校准失败，请重新校准！" "第二点校准失败，请重新校准！" "第三点校准失败，请重新校准！"] -> w954
              frame "第一点确认校准", Default {
              }
              frame "第二点确认校准" {
              }
              frame "第三点确认校准" {
              }
            }
            n497 = Equal?(x=w958, y=w957) -> (x = y?=w947:bool)
            n498 = Select(t="校准成功！", s=w947, f=w956) -> (s? t:f=w952:string)
            n499 = Select(t="校准失败！", s=w947, f=w954) -> (s? t:f=w951:string)
            n500 = Bundle By Name(cluster=errorcluster {"status"=FALSE, "code"=0, "source"="校准成功！"} ("error in (no error)"), "source"=w952) -> (w949:errorcluster)
            n501 = Bundle By Name(cluster=errorcluster {"status"=TRUE, "code"=0, "source"="校准失败！"} ("error in (no error)"), "source"=w951) -> (w948:errorcluster)
          }
        }
        n502 = property on="测量量程" class="Ring (strict)"() -> ("Value"=w903:u16)  [unwired: 2 in, 2 out]
        n503 = property on="标液一" class="Clust (strict)"() -> ("Value"=w915:cluster{"标准值":dbl, "检测值":dbl, "原始值":dbl})  [unwired: 2 in, 2 out]
        n504 = property on="标液二" class="Clust (strict)"() -> ("Value"=w914:cluster{"标准值":dbl, "检测值":dbl, "原始值":dbl})  [unwired: 2 in, 2 out]
        n505 = property on="标液三" class="Clust (strict)"() -> ("Value"=w913:cluster{"标准值":dbl, "检测值":dbl, "原始值":dbl})  [unwired: 2 in, 2 out]
        n506 = call "执行校准.vi"("校准点位"=w906, "校准方式"=w909, "校准量程"=w903, "校准参数"=w910, "标液三"=w913, "标液二"=w914, "标液一"=w915) -> ("error out"=w908:errorcluster)  [unwired: 4 in]
        n507 = case shown="No Error" w908 {
          selector: w908 -> [_ w940]
          tunnel: [w933 "校准失败！"] -> w916
          tunnel: [w934 w940] -> w907
          tunnel: w905 -> [w932 _]
          tunnel: w904 -> [w931 _]
          frame No Error {
            n508 = flat-sequence {
              tunnel: [w937] -> w935
              frame #0 {
                n509 = Wait (ms)(milliseconds to wait=u32 2000 ("等待时间（毫秒）")) -> ()  [unwired: 1 out]
              }
              frame #1 {
                n510 = property on="电极状态标志" class="DigNum (strict)"() -> ("Value"=w938:u16)  [unwired: 2 in, 2 out]
                n511 = case shown="0..2, 31..33" w938 {
                  tunnel: [_ TRUE] -> w937
                  frame Default {
                  }
                  frame 0..2, 31..33 {
                  }
                }
              }
            }
            n512 = Select(t=w932, s=w935, f=w931) -> (s? t:f=w934:errorcluster)
            n513 = Unbundle By Name(w934) -> ("source"=w933:string)
          }
          frame Error {
          }
        }
        n514 = One Button Dialog(message=w916) -> ()  [unwired: 1 in, 1 out]
        n515 = case shown="True" w911 {
          tunnel: w915 -> [_ w930]
          tunnel: w914 -> [_ w929]
          tunnel: w913 -> [_ w928]
          tunnel: w910 -> [_ w919]
          tunnel: w909 -> [_ w923]
          tunnel: w907 -> [_ w927]
          frame False {
          }
          frame True {
            n516 = call "探头测量值显示.vi"("校准参数"=w919) -> ("线性系数"=w922:cluster{bool, "K":sgl, "B":sgl})  [unwired: 3 in, 7 out]
            n517 = Unbundle By Name(w922) -> ("K"=w921:sgl, "B"=w920:sgl)
            n518 = control-ref of="校准记录"() -> (w925:refnum<vi>)
            n519 = property on="当前温度" class="DigNum (strict)"() -> ("Value"=w926:dbl)  [unwired: 2 in, 2 out]
            n520 = property on="序列号" class="Str"() -> ("Value"=w924:string)  [unwired: 2 in, 2 out]
            n521 = call "生成校准记录.vi"("标液一"=w930, "校准参数"=w919, "校准方式"=w923, "校准记录"=w925, "标液二"=w929, "标液三"=w928, "当前温度"=w926, "error in (no error)"=w927, "序列号"=w924, "K"=w921, "B"=w920) -> ()  [unwired: 3 in, 2 out]
          }
        }
      }
    }
  }
  n522 = while {
    tunnel: w1 -> [w972]
    stop <- FALSE stop-if-true
    n523 = Wait on Occurrence(2:w972) -> (0:w970:bool)  [unwired: 2 in]
    n524 = flat-sequence {
      tunnel: w970 -> [_]
      frame #0 {
        n525 = call "信号曲线.vi"() -> ()  [unwired: 12 in]
      }
    }
  }
  n526 = property on="窗格" class="Pane"("Origin"=T1 {"Horizontal"=0, "Vertical"=0} ("原点")) -> ()  [unwired: 2 in, 2 out]
